vi "MAIN.vi"() -> ()   [LabVIEW 2013]
uses:
  <vilib>/Utility/miscctls.llb/LVRectTypeDef.ctl
  <vilib>/DAQmx/write.llb/DAQmx Write (Analog DBL 1Chan 1Samp).vi
  <vilib>/DAQmx/read.llb/DAQmx Read (Analog 1D DBL NChan 1Samp).vi
  <vilib>/Utility/inputDevices.llb/closeJoystick.vi
  <vilib>/Utility/file.llb/Read From Spreadsheet File (string).vi
  <vilib>/Utility/file.llb/Read From Spreadsheet File (I64).vi
  <vilib>/DAQmx/miscellaneous.llb/DAQmx Fill In Error Info.vi
  <vilib>/Utility/inputDevices.llb/joystickAcquire.vi
panel:
  out "drift_correction_ref":dbl
  out "gpd present":bool
  in  "piezo move":bool=TRUE
  out "device index":i32
  out "read":i64[](array[numeric])
  out "chnl_control":enum16{"MAIN", "QUIT", "INIT", "SAVE"}(ring)=enum."INIT"
  out "state control":T1(ring)=enum."INIT"
  out "channels":string[](array[string])
  out "config":i32[](array[numeric])
  out "Est Power peak":dbl=2.5048715520372213e-09 format="%.4e"
  out "psd":dbl[](graph)
  out "PIEZO":dbl[](graph)
  out "gpd save":bool
  out "gpd start":bool
  out "Tab Control":enum32{"VELO", "KALIB", "channels", "gamepad"}(tab)
  out "Boolean 2":bool
  out "A+B+C+D":dbl format="%#_4f"
  out "(A+B)-(D+C)\n  A+B+C+D":dbl format="%#_4f"
  out "piezo \nposition [nm]":dbl format="%#_4f"
  in  "Z scansize [nm]":i64(slide)=10 min=6000 scale=0.0..6000.0
  in  "Z scanstart [nm]":i64(slide)=10 max=6000 scale=0.0..6000.0
  out "PSD RT":dbl(graph)
  out "first":cluster{"Best Polynomial Fit":dbl[], dbl[]}[](graph)
  in  "SAVE":bool
  in  "start":bool
  out "controls":enum32{"Main controls", "Sub controls"}(tab)
  in  "Advanced":bool
  in  "output folder":path
  in  "multiplier":dbl=10.0
  in  "Gamepad":bool
  in  "kalibruj":bool
  in  "exit":bool
  in  "pause":bool
  in  "slope [nm/V]":dbl format="%.5f"
  in  "pulling speed [nm/s]":dbl=400.0
  in  "Measure\n slope?":bool
  in  "accept calibration":bool
  out "pulling duration [s]":dbl
  in  "piezo movement":enum32{"Radio Selection 1", "Radio Selection 2"}(radio)
  in  "spring constant [N/m]":dbl format="%.5f"
  out "Force [pN]":dbl format="%.2f"
  out "Length [nm]":dbl format="%.2f"
  out "curves count":dbl
  out "saved curves count":i64
  in  "RT DEFLECTION CORRECTION":bool
  in  "deflection correction":bool=TRUE
  in  "alarm":bool=TRUE
  in  "Flip X":bool=TRUE
  in  "Flip Y":bool
  in  "piezo correction hysteresis window [nm]":u32=20
  in  "Drift_crr":bool
  in  "save defaults":bool
  in  "Basic":bool
  in  "spring constatnt\ncorrection factor":dbl=0.817
  in  "samples count/curve":dbl=10000.0 min=100.0 max=1000000.0 step=10000.0
  in  "bcfg":bool
  in  "Terminal_Config":bool
  in  "ambient temp. [Celsius]":dbl=22.0
  in  "auto interval [ms]":u32=1000 max=1000000 step=100
  in  "autosave":bool
  in  "automeasure count":dbl
  in  "auto":bool
  in  "to txt":bool=TRUE
  in  "to datalog":bool=TRUE
  in  "to punias":bool
  out "power peak":dbl
  in  "ponów":bool
  in  "koniec":bool
  in  "stop 2":bool
  in  "Averages":u32(slide)=128 min=64 max=1024 step=64 scale=64.0..1024.0
  out "Spectrum Plot":cluster{dbl, "df":dbl, "Spectrum out":dbl[]}(graph)
  in  "Sampling frequency [Hz]":dbl(slide)=100000.0 step=10000.0 scale=50000.0..150000.0 scale format="%#1_3p"
  in  "Boolean":bool
  in  "piezo sensitivity [nm/V]":dbl=1505.255 format="%#_13g"
  in  "maximum piezo movement range [nm]":i32=6000
  in  "ignore hw error":bool=TRUE
  out "path":path
  in  "SAVE 2":bool
  in  "RELOAD CONFIG":bool
  in  "QUIT":bool
  in  "PIEZO OUTPUT":tag
  in  "PIEZO INPUT":tag
  in  "[(A+B)-(C+D)]/(A+B+C+D)":tag
  in  "A+B+C+D":tag
  in  "gpd_confirm":bool
  in  "device_ok":bool
  out "device name":string
  in  "index":i32
  out "pov 2":bool
  out "pov 3":bool
  out "pov 4":bool
  out "pov 1":bool
  out "button 10":bool
  out "button 9":bool
  out "button 8":bool
  out "button 7":bool
  out "button 6":bool
  out "button 5":bool
  out "button 4":bool
  out "button 3":bool
  out "button 2":bool
  out "button 1":bool
  in  "Ring 14":u16(ring) items=["blank", "speed--", "speed++", "scanstart--", "scanstart++", "scansize--", "scansize++", "x1000", "x100", "x10", "save", "start"]
  in  "Ring 13":u16(ring) items=["blank", "speed--", "speed++", "scanstart--", "scanstart++", "scansize--", "scansize++", "x1000", "x100", "x10", "save", "start"]
  in  "Ring 12":u16(ring) items=["blank", "speed--", "speed++", "scanstart--", "scanstart++", "scansize--", "scansize++", "x1000", "x100", "x10", "save", "start"]
  in  "Ring 8":u16(ring) items=["blank", "speed--", "speed++", "scanstart--", "scanstart++", "scansize--", "scansize++", "x1000", "x100", "x10", "save", "start"]
  in  "Ring 9":u16(ring) items=["blank", "speed--", "speed++", "scanstart--", "scanstart++", "scansize--", "scansize++", "x1000", "x100", "x10", "save", "start"]
  in  "Ring 7":u16(ring) items=["blank", "speed--", "speed++", "scanstart--", "scanstart++", "scansize--", "scansize++", "x1000", "x100", "x10", "save", "start"]
  in  "Ring 11":u16(ring) items=["blank", "speed--", "speed++", "scanstart--", "scanstart++", "scansize--", "scansize++", "x1000", "x100", "x10", "save", "start"]
  in  "Ring 10":u16(ring) items=["blank", "speed--", "speed++", "scanstart--", "scanstart++", "scansize--", "scansize++", "x1000", "x100", "x10", "save", "start"]
  in  "Ring 2":u16(ring) items=["blank", "speed--", "speed++", "scanstart--", "scanstart++", "scansize--", "scansize++", "x1000", "x100", "x10", "save", "start"]
  in  "Ring 4":u16(ring) items=["blank", "speed--", "speed++", "scanstart--", "scanstart++", "scansize--", "scansize++", "x1000", "x100", "x10", "save", "start"]
  in  "Ring 6":u16(ring) items=["blank", "speed--", "speed++", "scanstart--", "scanstart++", "scansize--", "scansize++", "x1000", "x100", "x10", "save", "start"]
  in  "Ring 3":u16(ring) items=["blank", "speed--", "speed++", "scanstart--", "scanstart++", "scansize--", "scansize++", "x1000", "x100", "x10", "save", "start"]
  in  "Ring 5":u16(ring) items=["blank", "speed--", "speed++", "scanstart--", "scanstart++", "scansize--", "scansize++", "x1000", "x100", "x10", "save", "start"]
  in  "Ring":u16(ring) items=["blank", "speed--", "speed++", "scanstart--", "scanstart++", "scansize--", "scansize++", "x1000", "x100", "x10", "save", "start"]
  out "appended array":bool[](array[boolean])
  # "K.Pawlak, J.Strzelecki, Institute of Physics, Nicolaus Copernicus University, Toruñ, Poland"
  # "setup settings"
  # "auto settings"
  # "save formats"
  # "curve"
  # "TERMINAL CONFIGURATION"
  # "1. SELECT PROPER DEVICE"
  # "PREVIEW"
  # "blank\nspeed--\nspeed++\nscanstart--\nscanstart++\nscansize--\nscansize++\nx1000\nx100\nx10\nsave\nstart"
  # "2. CHOOSE BUTTONS FUNCTIONS"
  # "3. CONFIRM BUTTON SETUP"
  # "author K.Pawlak\nInstitute of Physics\nNicolaus Copernicus University\nToruñ, Poland\nAFM gamepad config. ver. 1.0"
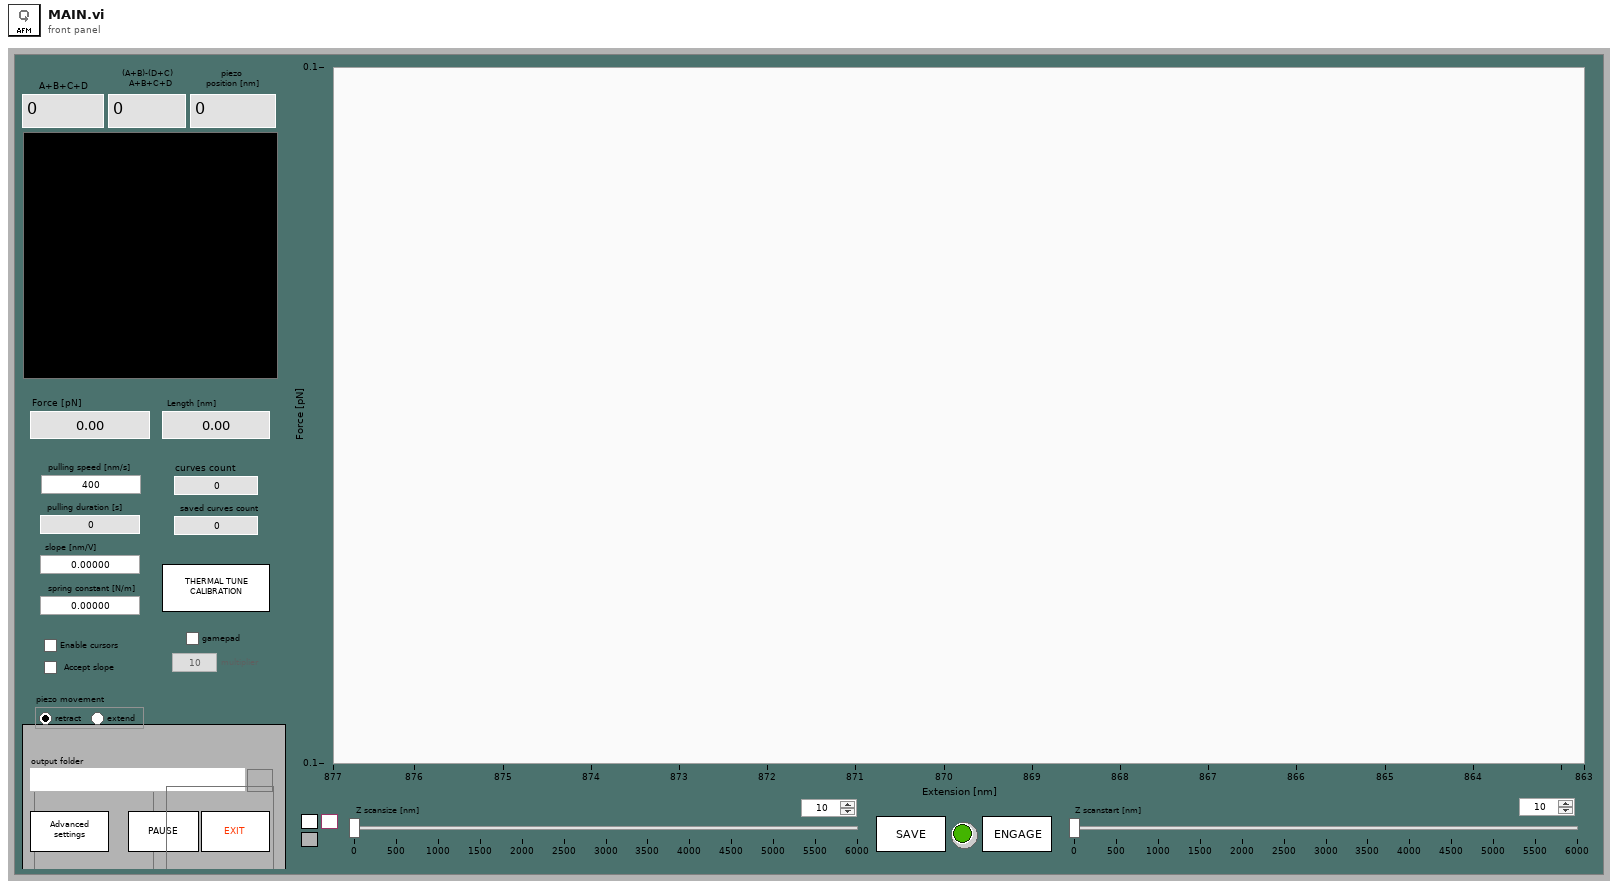
[diagram p1: front panel]
types:
  T1 = enum16{"kalibracja", "INIT", "2", "SAVE", "IDLE", "channels", "pad_cfg"}
  T2 = enum16{"open", "replace", "create", "open or create", "replace or create", "replace or create with confirmation"}
  T3 = enum8{"Enabled", "Disabled", "Disabled and Grayed Out"}
  T4 = typedef "LVRectTypeDef.ctl" = cluster{"Left":i16, "Top":i16, "Right":i16, "Bottom":i16}
  T5 = enum32{"Invalid", "Standard", "Closed", "Hidden", "Minimized", "Maximized"}
  T6 = enum16{"kalibracja", "INIT", "2", "SAVE", "IDLE", "channels"}
  T7 = enum16{"kalibracja", "INIT", "2", "SAVE", "IDLE"}
  T8 = cluster{"PIEZO":dbl[], "psd":dbl[], "Z scanstart [nm]":i64, "slope [nm/V]":dbl, "spring constant [N/m]":dbl, "pulling speed [nm/s]":dbl, "time string":string}
  T9 = cluster{"axes total":u32, "buttons total":u32, "pov total":u32, "device name":string}[]
  T10 = cluster{"axes total":u32, "buttons total":u32, "pov total":u32, "device name":string}
  T11 = cluster{"button 1":bool, "button 2":bool, "button 3":bool, "button 4":bool, "button 5":bool, "button 6":bool, "button 7":bool, "button 8":bool, "button 9":bool, "button 10":bool, "button 11":bool, "button 12":bool, "button 13":bool, "button 14":bool, "button 15":bool, "button 16":bool, "button 17":bool, "button 18":bool, "button 19":bool, "button 20":bool, "button 21":bool, "button 22":bool, "button 23":bool, "button 24":bool, "button 25":bool, "button 26":bool, "button 27":bool, "button 28":bool, "button 29":bool, "button 30":bool, "button 31":bool, "button 32":bool}
  T12 = cluster{"pov 1":i32, "pov 2":i32, "pov 3":i32, "pov 4":i32}
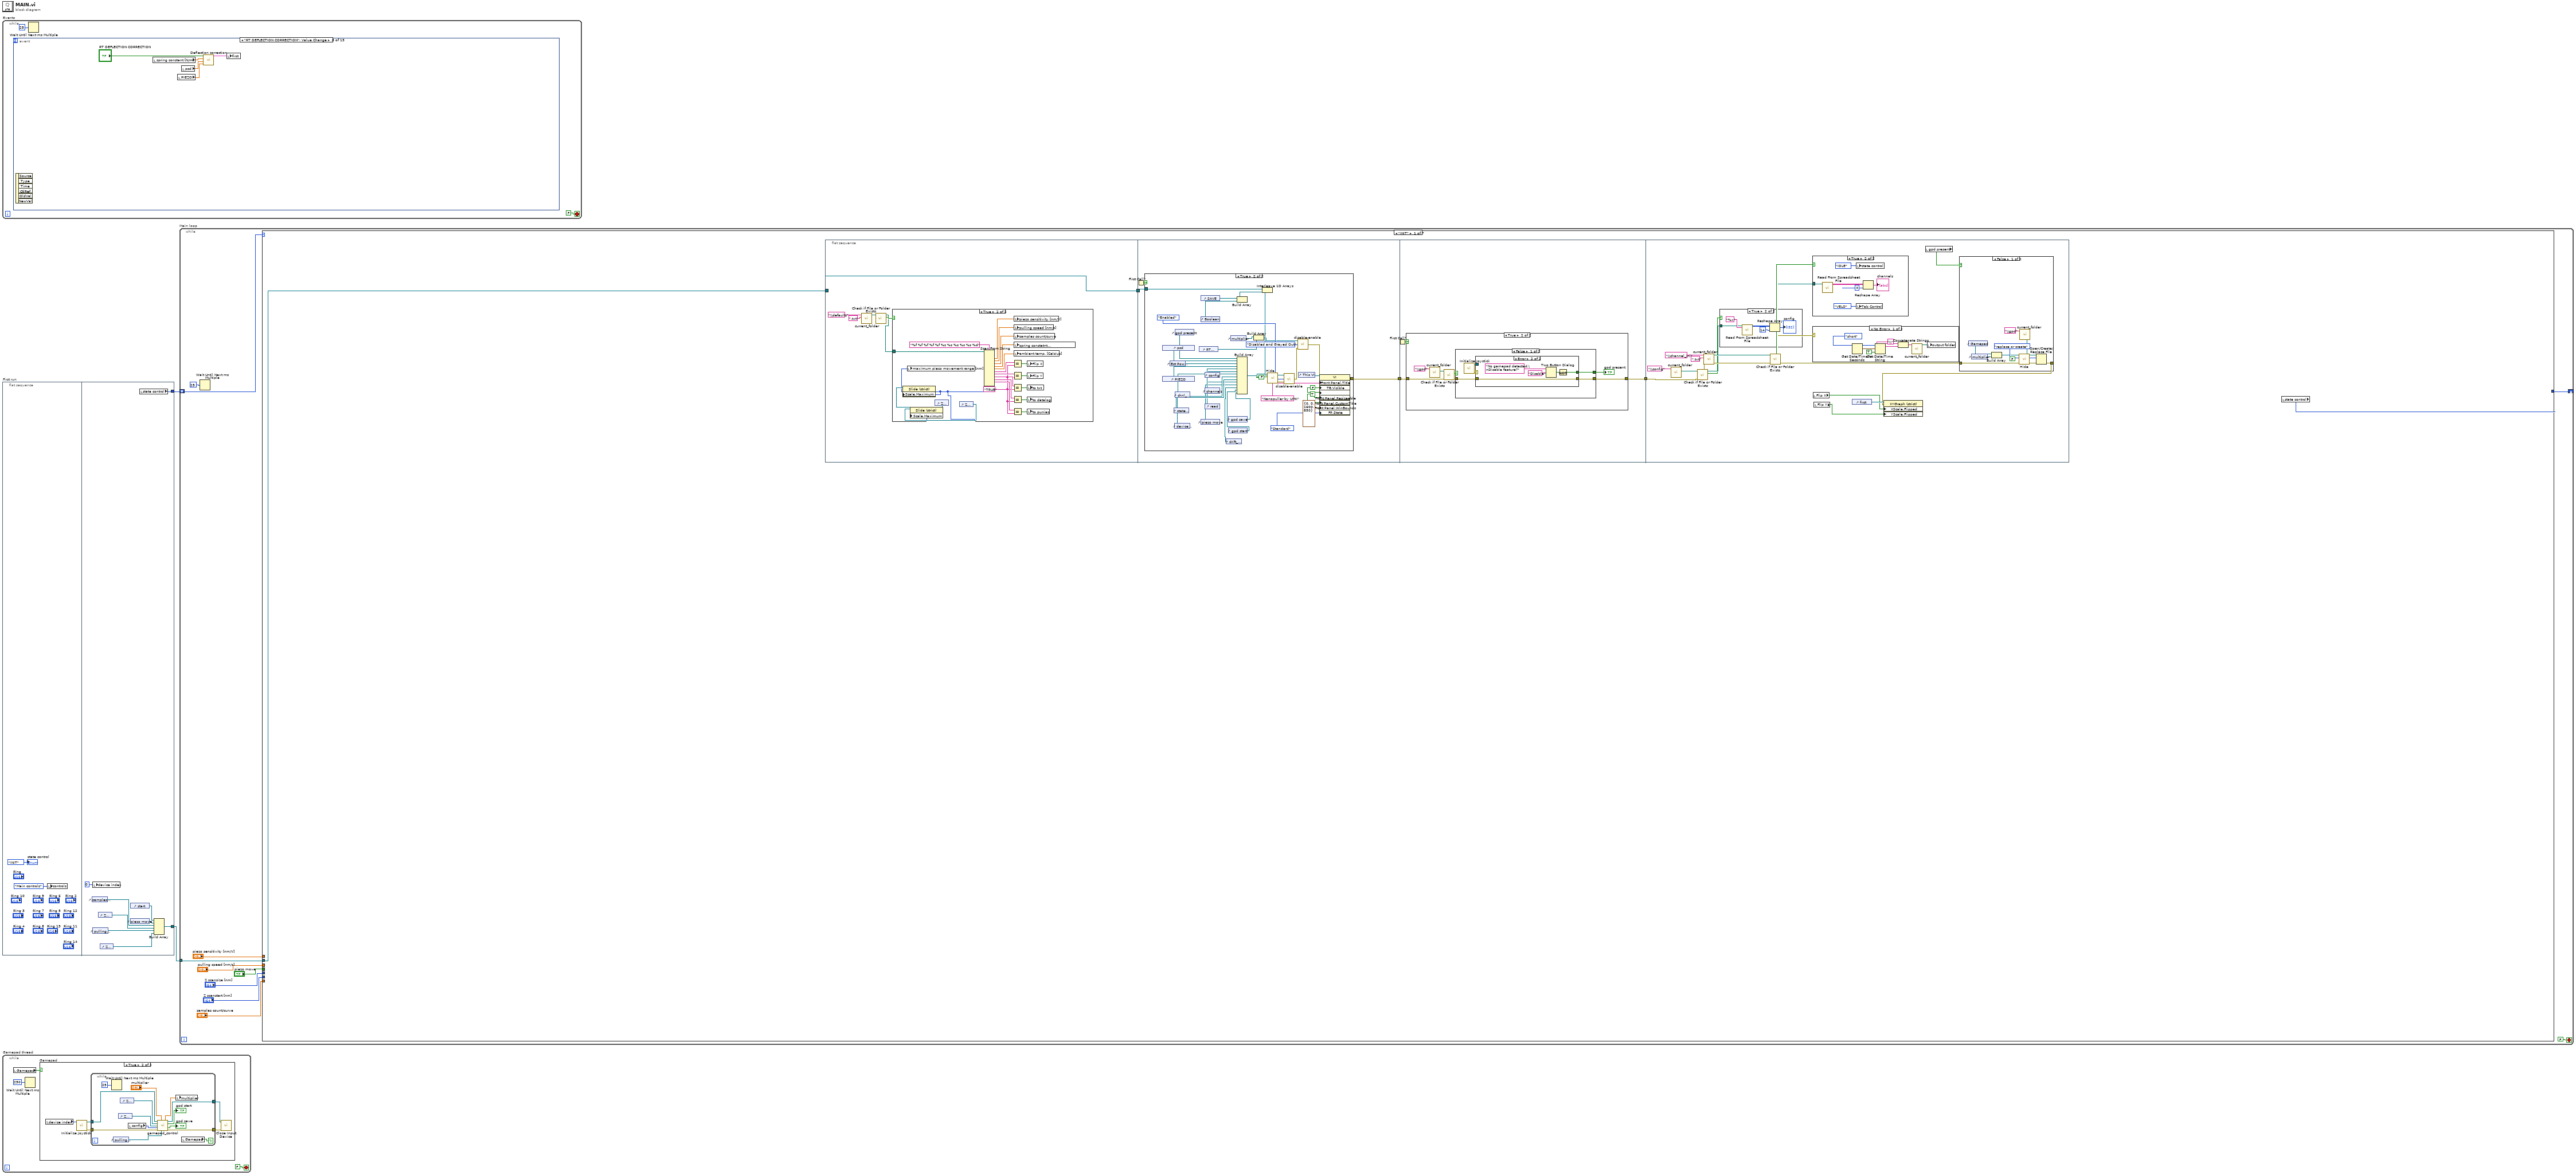
[diagram p0: block diagram]
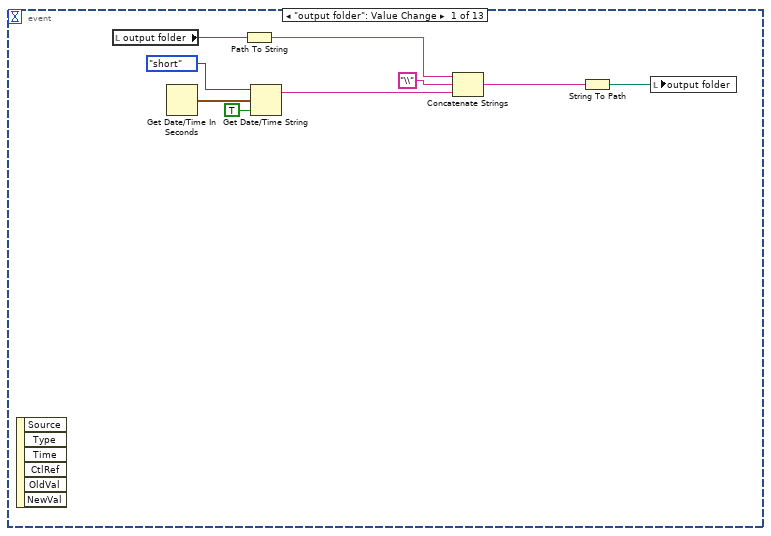
[diagram p3: hidden frame]
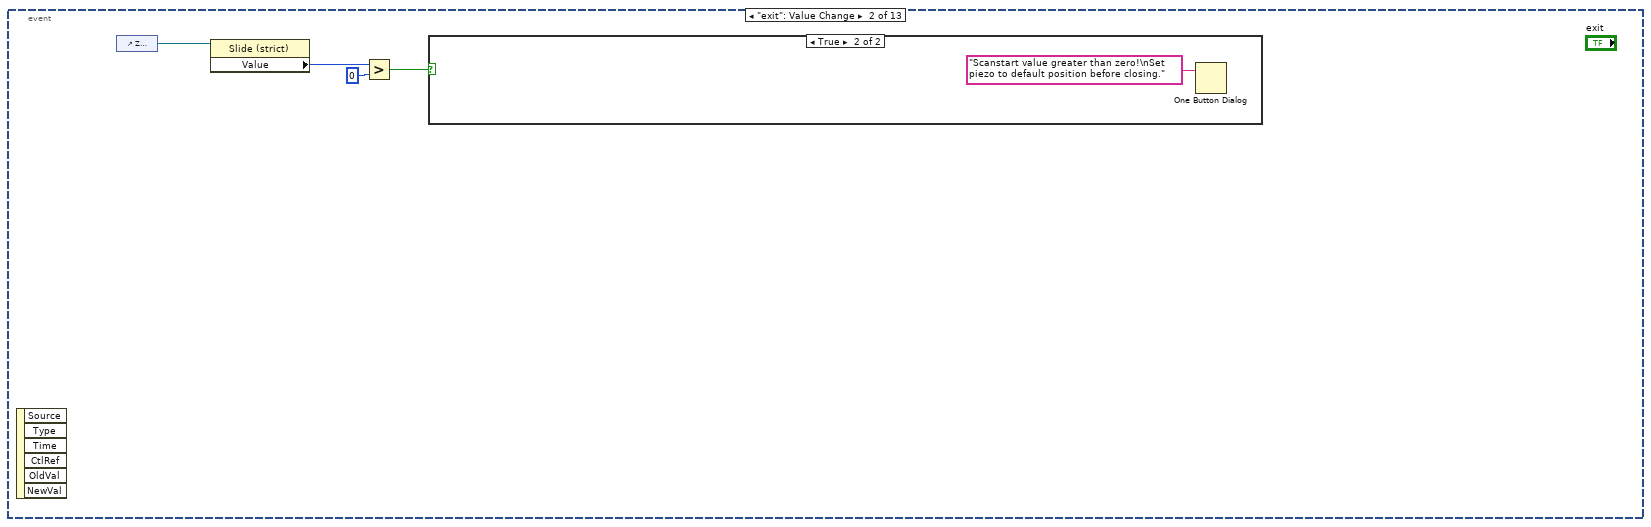
[diagram p4: hidden frame]
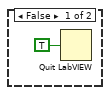
[diagram p5: hidden frame]
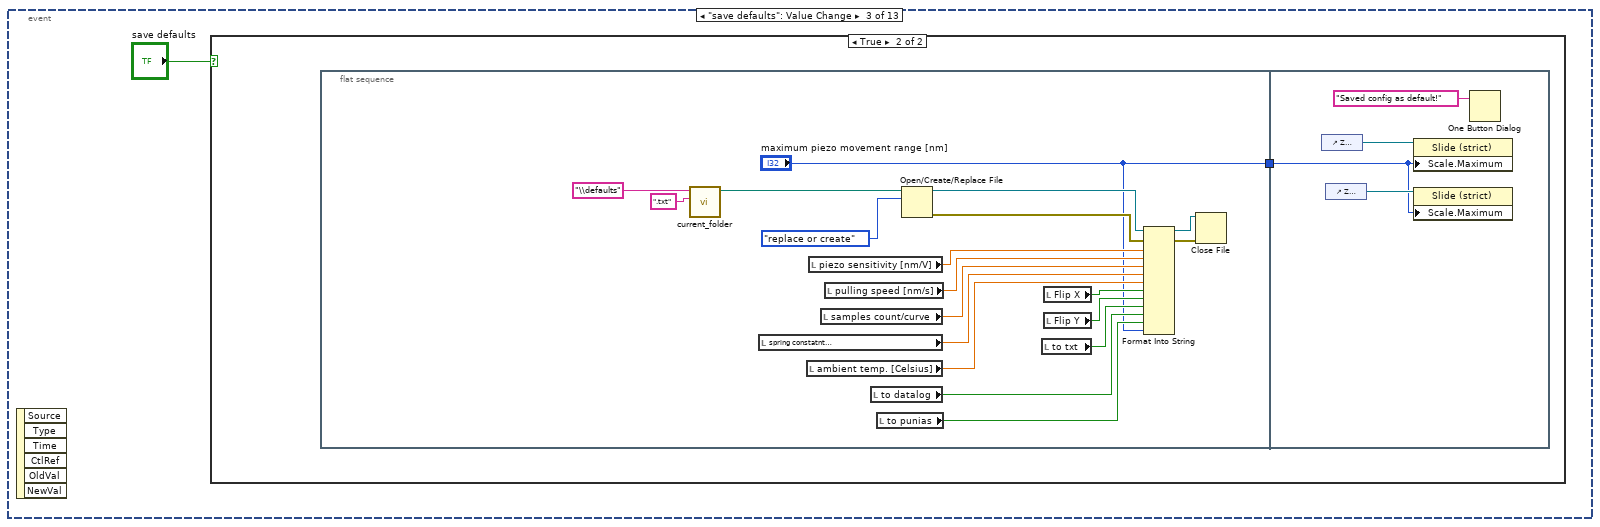
[diagram p6: hidden frame]
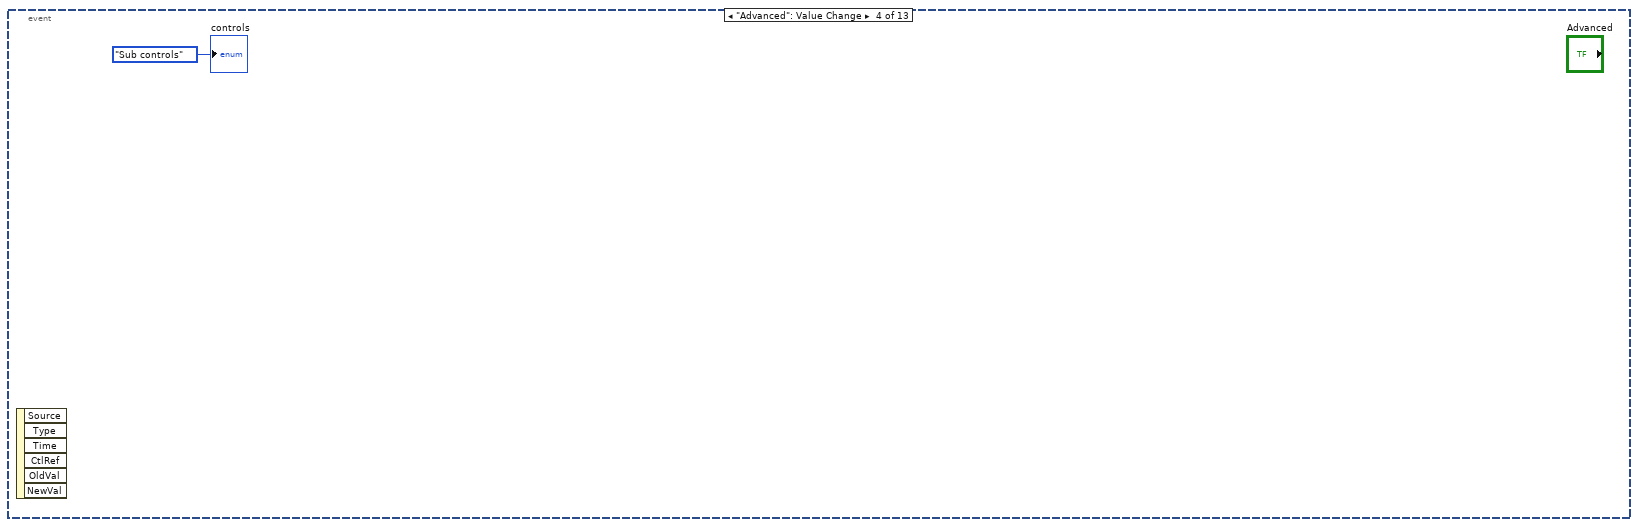
[diagram p8: hidden frame]
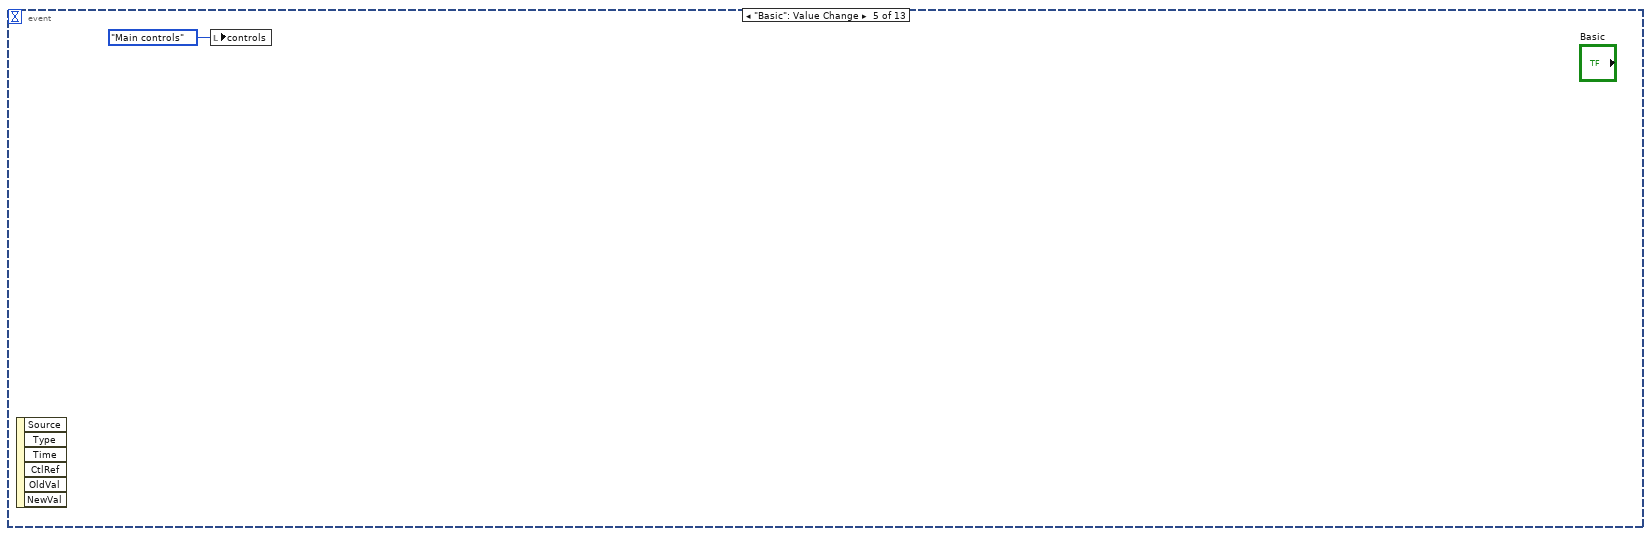
[diagram p9: hidden frame]
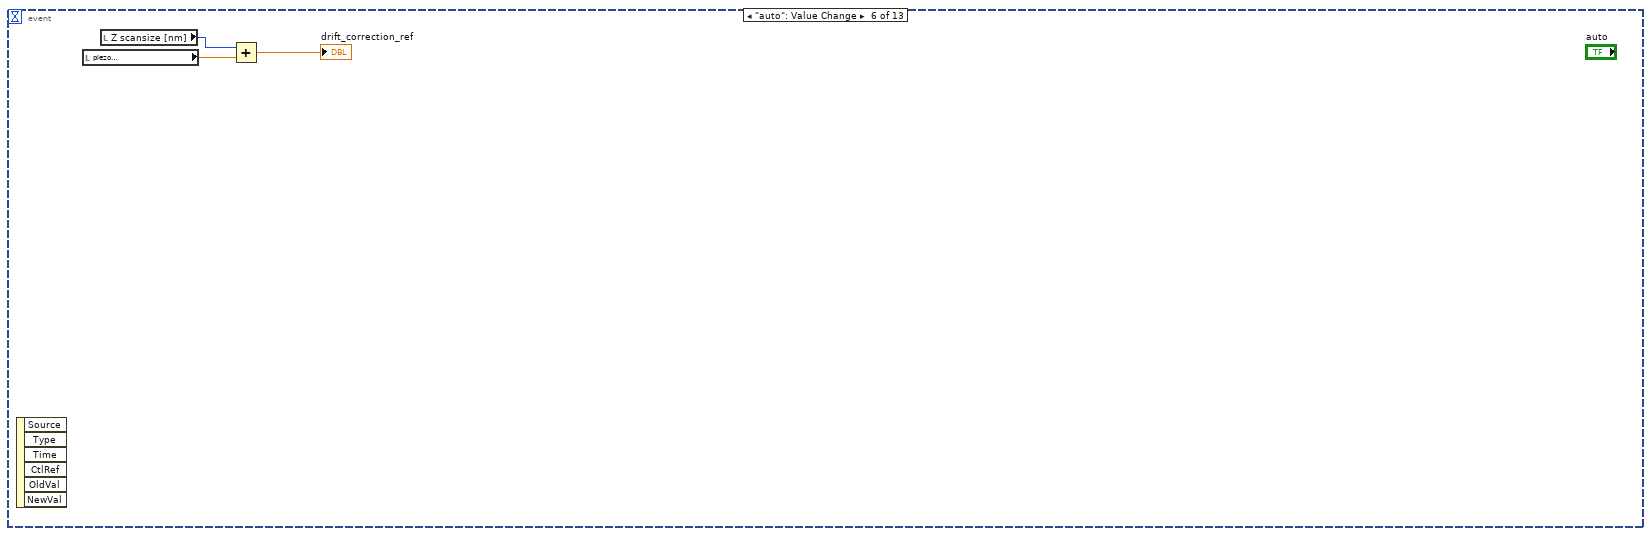
[diagram p10: hidden frame]
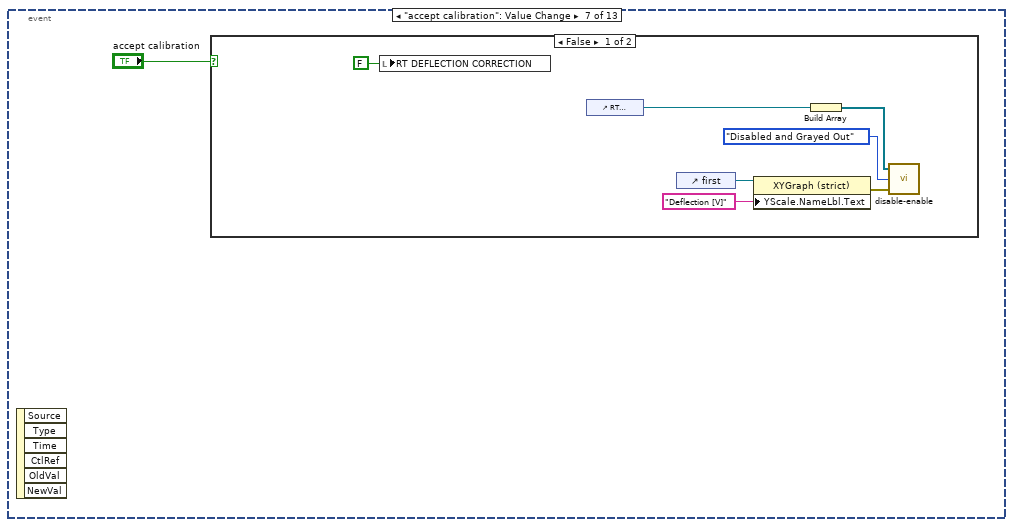
[diagram p11: hidden frame]
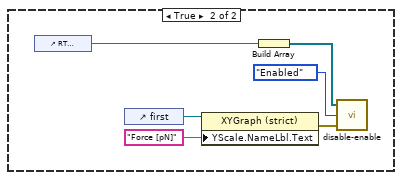
[diagram p12: hidden frame]
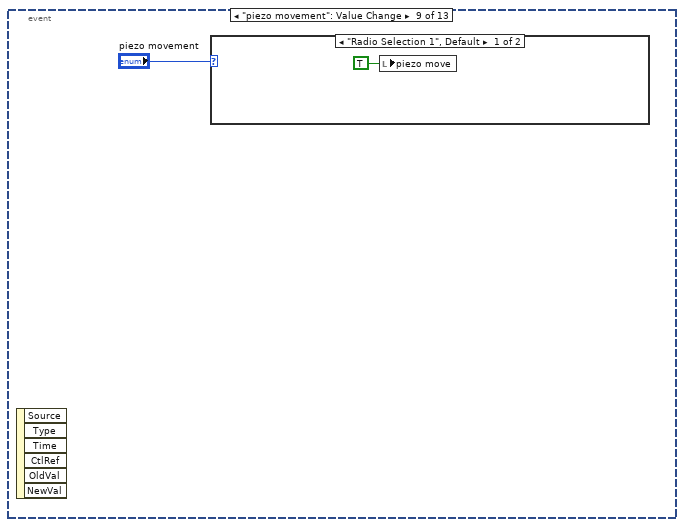
[diagram p13: hidden frame]
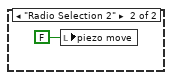
[diagram p14: hidden frame]
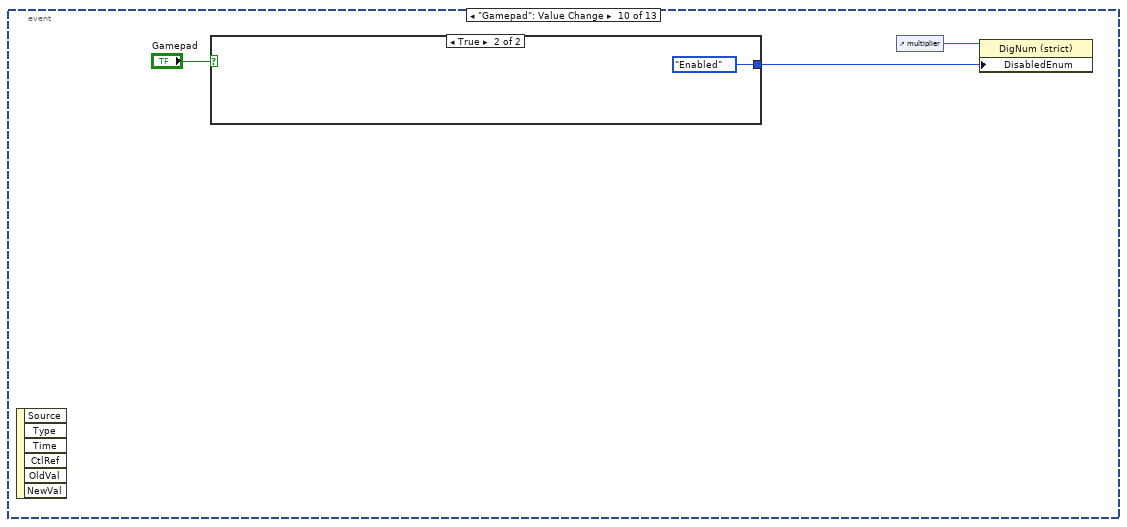
[diagram p15: hidden frame]
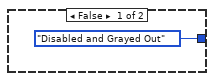
[diagram p16: hidden frame]
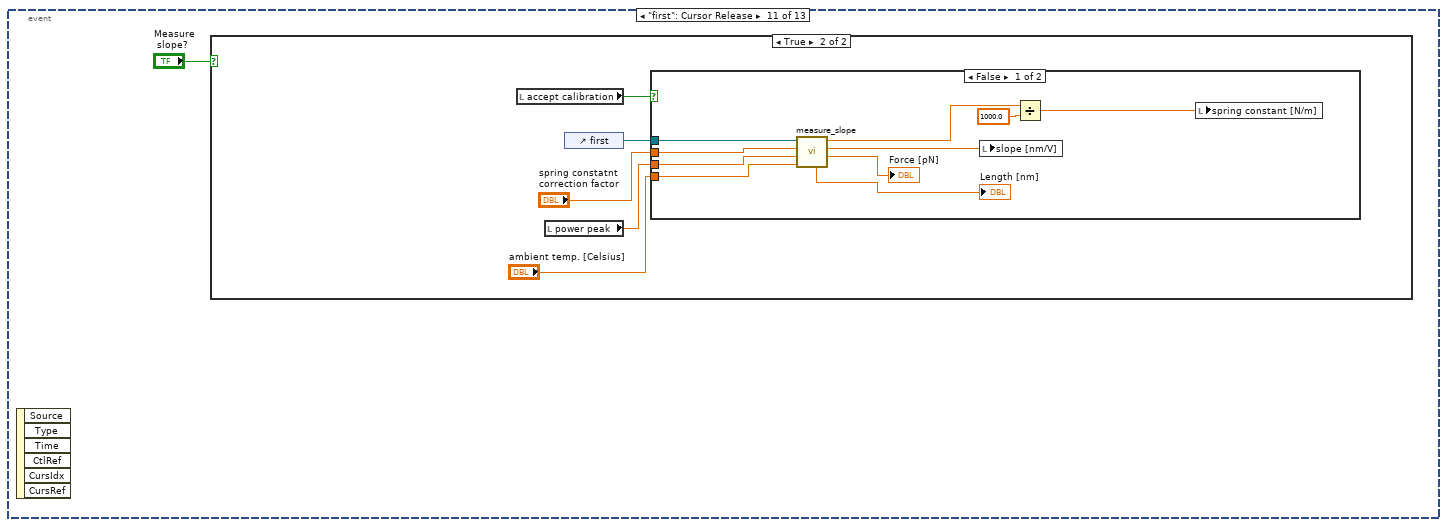
[diagram p17: hidden frame]
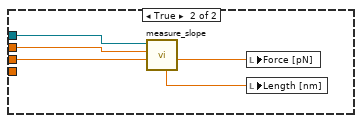
[diagram p19: hidden frame]
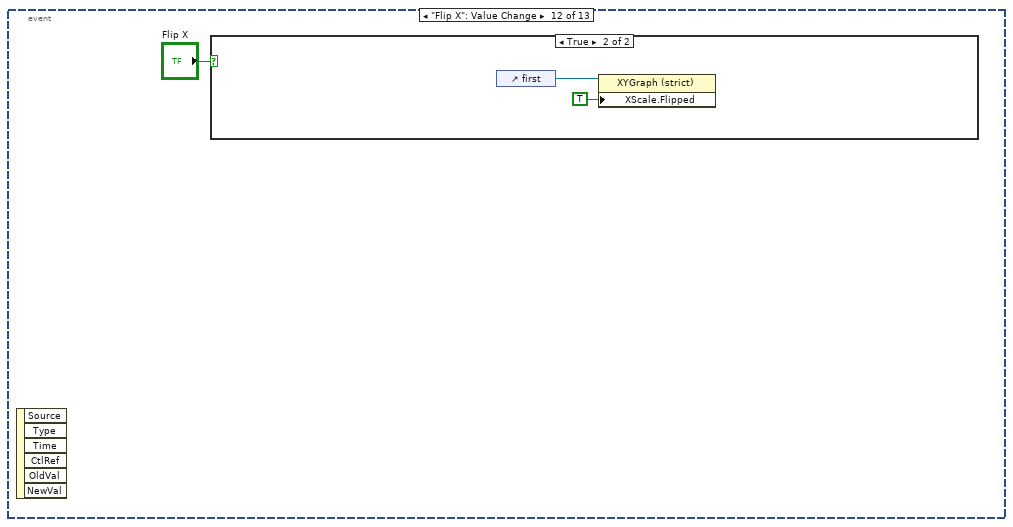
[diagram p20: hidden frame]
diagram:
  n1 = while "Events" {
    stop <- FALSE stop-if-true
    n2 = event shown="[7] \"RT DEFLECTION CORRECTION\": Value Change" {
      selector: _ -> [_ _ _ _ _ _ _ _ _ _ _ _ _]
      dyn-events: _ -> [_ _ _ _ _ _ _ _ _ _ _ _ _]
      timeout: _ -> [_ _ _ _ _ _ _ _ _ _ _ _ _]
      event "output folder": Value Change {
        n3 = event-data() -> ()  [unwired: 1 in, 6 out]
        n4 = local read "output folder"() -> (w10:path)
        n5 = Get Date/Time In Seconds() -> (seconds since 1Jan1904=w12:timestamp)
        n6 = Path To String(path=w10) -> (string=w9:string)
        n7 = Get Date/Time String(date format (0)=enum16{"short", "long", "abbreviated"}."short", seconds (now)=w12, want seconds? (F)=TRUE) -> (date string=w6:string)  [unwired: 1 out]
        n8 = Concatenate Strings(w9, "\\" ("string"), w6) -> (w7:string)
        n9 = String To Path(string=w7) -> (path=w8:path)
        n10 = local write "output folder"(w8) -> ()
      }
      event "exit": Value Change {
        n11 = event-data() -> ()  [unwired: 1 in, 6 out]
        n12 = control-ref of="Z scanstart [nm]"() -> (w15:refnum<vi>)
        n13 = property class="Slide (strict)"(reference=w15) -> ("Value"=w16:i64)  [unwired: 1 in, 2 out]
        n14 = Greater?(x=w16, y=i64 0) -> (0:w14:bool)
        n15 = case shown="True" w14 {
          frame False {
            n16 = Quit LabVIEW(quit? (T)=TRUE) -> ()
          }
          frame True {
            n17 = One Button Dialog(message="Scanstart value greater than zero!\nSet piezo to default position before closing.") -> ()  [unwired: 1 in, 1 out]
          }
        }
      }
      event "save defaults": Value Change {
        n18 = event-data() -> ()  [unwired: 1 in, 6 out]
        n19 = case shown="True" "save defaults" {
          frame False {
          }
          frame True {
            n20 = flat-sequence {
              tunnel: ["maximum piezo movement range [nm]"] -> w21
              tunnel: w21 -> [w41]
              frame #0 {
                n21 = call "current_folder.vi"("extension"=".txt", "filename"="\\defaults") -> ("Path"=w30:path)  [unwired: 9 in]
                n22 = local read "spring constatnt\ncorrection factor"() -> (w33:dbl)
                n23 = local read "ambient temp. [Celsius]"() -> (w32:dbl)
                n24 = local read "piezo sensitivity [nm/V]"() -> (w36:dbl)
                n25 = local read "samples count/curve"() -> (w34:dbl)
                n26 = local read "pulling speed [nm/s]"() -> (w35:dbl)
                n27 = local read "to datalog"() -> (w24:bool)
                n28 = local read "to punias"() -> (w23:bool)
                n29 = Open/Create/Replace File(file path (use dialog)=w30, operation (0:open)=T2."replace or create") -> (refnum out=w29:refnum<file>, error out=w26:errorcluster)  [unwired: 4 in, 1 out]
                n30 = local read "to txt"() -> (w25:bool)
                n31 = local read "Flip X"() -> (w39:bool)
                n32 = local read "Flip Y"() -> (w38:bool)
                n33 = Format Into String(initial string=w29, error in=w26, w36, w35, w34, w33, w32, w39, w38, w25, w24, w23, "maximum piezo movement range [nm]") -> (resulting string=w28:refnum<file>, error out=w27:errorcluster)  [unwired: 1 in]
                n34 = Close File(refnum=w28, error in=w27) -> ()  [unwired: 2 out]
              }
              frame #1 {
                n35 = control-ref of="Z scanstart [nm]"() -> (w42:refnum<vi>)
                n36 = control-ref of="Z scansize [nm]"() -> (w43:refnum<vi>)
                n37 = property class="Slide (strict)"(reference=w42, "Scale.Maximum"=w41) -> ()  [unwired: 1 in, 2 out]
                n38 = property class="Slide (strict)"(reference=w43, "Scale.Maximum"=w41) -> ()  [unwired: 1 in, 2 out]
                n39 = One Button Dialog(message="Saved config as default!") -> ()  [unwired: 1 in, 1 out]
              }
            }
          }
        }
      }
      event "Advanced": Value Change {
        n40 = event-data() -> ()  [unwired: 1 in, 6 out]
        "controls" <- enum32{"Main controls", "Sub controls"}."Sub controls" ("controls")
      }
      event "Basic": Value Change {
        n41 = event-data() -> ()  [unwired: 1 in, 6 out]
        n42 = local write "controls"(enum32{"Main controls", "Sub controls"}."Main controls" ("controls")) -> ()
      }
      event "auto": Value Change {
        n43 = event-data() -> ()  [unwired: 1 in, 6 out]
        n44 = local read "piezo \nposition [nm]"() -> (w48:dbl)
        n45 = local read "Z scansize [nm]"() -> (w49:i64)
        n46 = Add(x=w49, y=w48) -> (x+y=→"drift_correction_ref":dbl)
      }
      event "accept calibration": Value Change {
        n47 = event-data() -> ()  [unwired: 1 in, 6 out]
        n48 = case shown="False" "accept calibration" {
          frame False {
            n49 = local write "RT DEFLECTION CORRECTION"(FALSE ("RT DEFLECTION CORRECTION")) -> ()
            n50 = control-ref of="RT DEFLECTION CORRECTION"() -> (w55:refnum<vi>)
            n51 = control-ref of="first"() -> (w57:refnum<vi>)
            n52 = property class="XYGraph (strict)"(reference=w57, "YScale.NameLbl.Text"="Deflection [V]" ("X Scale.Name Label.Text")) -> (error out=w52:errorcluster)  [unwired: 1 in, 1 out]
            n53 = Build Array(w55) -> (w54:refnum<vi>[])
            n54 = call "disable-enable.vi"("error in (no error)"=w52, "Disabled"=T3."Disabled and Grayed Out", "Array"=w54) -> ()  [unwired: 1 out]
          }
          frame True {
            n55 = control-ref of="RT DEFLECTION CORRECTION"() -> (w61:refnum<vi>)
            n56 = control-ref of="first"() -> (w63:refnum<vi>)
            n57 = property class="XYGraph (strict)"(reference=w63, "YScale.NameLbl.Text"="Force [pN]" ("X Scale.Name Label.Text")) -> (error out=w58:errorcluster)  [unwired: 1 in, 1 out]
            n58 = Build Array(w61) -> (w60:refnum<vi>[])
            n59 = call "disable-enable.vi"("error in (no error)"=w58, "Disabled"=T3."Enabled", "Array"=w60) -> ()  [unwired: 1 out]
          }
        }
      }
      event "RT DEFLECTION CORRECTION": Value Change {
        n60 = event-data() -> ()  [unwired: 1 in, 6 out]
        n61 = local read "spring constant [N/m]"() -> (w67:dbl)
        n62 = local read "PIEZO"() -> (w65:dbl[])
        n63 = local read "psd"() -> (w66:dbl[])
        n64 = call "Deflection correction.vi"("fitted piezo"=w65, "psd"=w66, "spring constant [N/m]"=w67, "RT DEFLECTION CORRECTION"="RT DEFLECTION CORRECTION") -> ("Array"=w64:cluster{dbl[], dbl[]}[])  [unwired: 7 in]
        n65 = local write "first"(w64) -> ()
      }
      event "piezo movement": Value Change {
        n66 = event-data() -> ()  [unwired: 1 in, 6 out]
        n67 = case shown="\"Radio Selection 1\", Default" "piezo movement" {
          frame "Radio Selection 1", Default {
            n68 = local write "piezo move"(TRUE ("piezo move")) -> ()
          }
          frame "Radio Selection 2" {
            n69 = local write "piezo move"(FALSE ("piezo move")) -> ()
          }
        }
      }
      event "Gamepad": Value Change {
        n70 = event-data() -> ()  [unwired: 1 in, 6 out]
        n71 = case shown="True" "Gamepad" {
          tunnel: [T3."Disabled and Grayed Out" ("Disabled") T3."Enabled" ("Disabled")] -> w73
          frame False {
          }
          frame True {
          }
        }
        n72 = control-ref of="multiplier"() -> (w74:refnum<vi>)
        n73 = property class="DigNum (strict)"(reference=w74, "DisabledEnum"=w73) -> ()  [unwired: 1 in, 2 out]
      }
      event "first": Cursor Release {
        n74 = event-data() -> ()  [unwired: 1 in, 6 out]
        n75 = case shown="True" "Measure\n slope?" {
          frame False {
          }
          frame True {
            n76 = local read "accept calibration"() -> (w79:bool)
            n77 = local read "power peak"() -> (w80:dbl)
            n78 = control-ref of="first"() -> (w82:refnum<vi>)
            n79 = case shown="False" w79 {
              tunnel: w82 -> [w92 w95]
              tunnel: "spring constatnt\ncorrection factor" -> [w91 w94]
              tunnel: w80 -> [w90 w93]
              tunnel: "ambient temp. [Celsius]" -> [w85 _]
              frame False {
                n80 = call "measure_slope.vi"("temp"=w85, "power peak"=w90, "correction factor"=w91, "XYGraph in"=w92) -> ("Numeric 3"=→"Force [pN]":dbl, "Numeric 2"=w84:dbl, "Numeric"=w86:dbl, "Numeric 4"=→"Length [nm]":dbl)  [unwired: 4 in]
                n81 = local write "slope [nm/V]"(w84) -> ()
                n82 = Divide(x=w86, y=1000.0) -> (x/y=w83:dbl)
                n83 = local write "spring constant [N/m]"(w83) -> ()
              }
              frame True {
                n84 = call "measure_slope.vi"("power peak"=w93, "correction factor"=w94, "XYGraph in"=w95) -> ("Numeric 3"=w97:dbl, "Numeric 4"=w96:dbl)  [unwired: 5 in, 2 out]
                n85 = local write "Force [pN]"(w97) -> ()
                n86 = local write "Length [nm]"(w96) -> ()
              }
            }
          }
        }
      }
      event "Flip X": Value Change {
        n87 = event-data() -> ()  [unwired: 1 in, 6 out]
        n88 = case shown="True" "Flip X" {
          frame False {
            n89 = control-ref of="first"() -> (w100:refnum<vi>)
            n90 = property class="XYGraph (strict)"(reference=w100, "XScale.Flipped"=FALSE ("X Scale.Flipped")) -> ()  [unwired: 1 in, 2 out]
          }
          frame True {
            n91 = control-ref of="first"() -> (w102:refnum<vi>)
            n92 = property class="XYGraph (strict)"(reference=w102, "XScale.Flipped"=TRUE ("X Scale.Flipped")) -> ()  [unwired: 1 in, 2 out]
          }
        }
      }
      event "Flip Y": Value Change {
        n93 = event-data() -> ()  [unwired: 1 in, 6 out]
        n94 = case shown="False" "Flip Y" {
          frame False {
            n95 = control-ref of="first"() -> (w105:refnum<vi>)
            n96 = property class="XYGraph (strict)"(reference=w105, "YScale.Flipped"=FALSE ("Y Scale.Flipped")) -> ()  [unwired: 1 in, 2 out]
          }
          frame True {
            n97 = control-ref of="first"() -> (w107:refnum<vi>)
            n98 = property class="XYGraph (strict)"(reference=w107, "YScale.Flipped"=TRUE ("Y Scale.Flipped")) -> ()  [unwired: 1 in, 2 out]
          }
        }
      }
    }
    n99 = Wait Until Next ms Multiple(millisecond multiple=u32 25) -> ()  [unwired: 1 out]
  }
  n100 = flat-sequence "First run" {
    tunnel: [w112] -> w2
    tunnel: [w111] -> w1
    frame #0 {
      n101 = local write "controls"(enum32{"Main controls", "Sub controls"}."Main controls" ("controls")) -> ()
      "state control" <- T1."INIT" ("state control")
    }
    frame #1 {
      n102 = control-ref of="samples count/curve"() -> (w115:refnum<vi>)
      n103 = control-ref of="pulling speed [nm/s]"() -> (w117:refnum<vi>)
      n104 = local write "device index"(0 ("device index")) -> ()
      n105 = control-ref of="Z scanstart [nm]"() -> (w116:refnum<vi>)
      n106 = control-ref of="Z scansize [nm]"() -> (w118:refnum<vi>)
      n107 = control-ref of="start"() -> (w113:refnum<vi>)
      n108 = control-ref of="piezo move"() -> (w114:refnum<vi>)
      n109 = local read "state control"() -> (w111:T1)
      n110 = Build Array(w113, w114, w115, w116, w117, w118) -> (w112:refnum<vi>[])
    }
  }
  n111 = while "Gamepad thread" {
    stop <- FALSE stop-if-true
    n112 = local read "Gamepad"() -> (w121:bool)
    n113 = Wait Until Next ms Multiple(millisecond multiple=u32 250) -> ()  [unwired: 1 out]
    n114 = case "Gamepad" shown="True" w121 {
      frame False {
      }
      frame True {
        n115 = local read "device index"() -> (w123:i32)
        n116 = call <vilib>:"Initialize Joystick.vi"("device index"=w123) -> ("error out"=w122:errorcluster, "device ID"=w126:refnum<k1>)  [unwired: 9 in]
        n117 = while {
          tunnel: w122 -> [w130]
          tunnel: w126 -> [w129]
          tunnel: [w128] -> w125
          tunnel: [w127] -> w124
          stop <- w134 continue-if-true
          n118 = Wait Until Next ms Multiple(millisecond multiple=u32 25) -> ()  [unwired: 1 out]
          n119 = control-ref of="pulling speed [nm/s]"() -> (w136:refnum<vi>)
          n120 = control-ref of="Z scanstart [nm]"() -> (w139:refnum<vi>)
          n121 = control-ref of="Z scansize [nm]"() -> (w140:refnum<vi>)
          n122 = local read "config"() -> (w135:i32[])
          n123 = call "gamepad_control.vi"("device ID in"=w129, "preskaler 2"="multiplier", "scansize [nm]"=w140, "scanstart [nm]"=w139, "read"=w135, "error in (no error)"=w130, "dynamika [nm/s]"=w136) -> ("preskaler"=w137:dbl, "Refnum out"=w128:refnum<k1>, "START"=→"gpd start":bool, "SAVE"=→"gpd save":bool, "error out"=w127:errorcluster)  [unwired: 3 in, 1 out]
          n124 = local write "multiplier"(w137) -> ()
          n125 = local read "Gamepad"() -> (w134:bool)
        }
        n126 = call-poly <vilib>:"Close Input Device.vi"("error in (no error)"=w124, "device ID"=w125) -> ()  [unwired: 8 in, 1 out]
      }
    }
  }
  n127 = while "Main loop" {
    tunnel: w2 -> [w151]
    shift-right: [w144] -> _
    shift-left: w1 -> [w145]
    stop <- FALSE stop-if-true
    n128 = Wait Until Next ms Multiple(millisecond multiple=u32 25 ("milliseconds to wait")) -> ()  [unwired: 1 out]
    n129 = case shown="\"INIT\"" w145 {
      tunnel: w151 -> [w156 w327 _ w550 _ _ _]
      tunnel: "Z scansize [nm]" -> [_ _ _ w552 _ _ _]
      tunnel: "pulling speed [nm/s]" -> [_ _ _ w548 _ _ _]
      tunnel: "Z scanstart [nm]" -> [_ _ _ w549 _ _ _]
      tunnel: "samples count/curve" -> [_ _ _ w547 _ _ _]
      tunnel: "piezo move" -> [_ _ _ w551 _ _ _]
      tunnel: [w155 w313 T7."IDLE" ("Enum 2") w546 w610 T1."INIT" ("state control") w891] -> w144
      tunnel: "piezo sensitivity [nm/V]" -> [_ w326 _ w545 _ _ _]
      frame "INIT" {
        n130 = flat-sequence {
          tunnel: w156 -> [w162]
          tunnel: [w162] -> w152
          tunnel: [w194] -> w154
          tunnel: w152 -> [w195]
          tunnel: w154 -> [w233]
          tunnel: [w232] -> w153
          tunnel: w153 -> [w265]
          frame #0 {
            n131 = call "current_folder.vi"("extension"=".txt", "filename"="\\defaults") -> ("Path"=w159:path)  [unwired: 9 in]
            n132 = call <vilib>:"Check if File or Folder Exists.vi"("path"=w159) -> ("file or folder exists?"=w158:bool, "dup path"=w157:path)  [unwired: 8 in, 1 out]
            n133 = case shown="True" w158 {
              tunnel: w157 -> [_ w187]
              frame False {
                n134 = control-ref of="ambient temp. [Celsius]"() -> (w165:refnum<vi>)
                n135 = control-ref of="piezo sensitivity [nm/V]"() -> (w170:refnum<vi>)
                n136 = control-ref of="samples count/curve"() -> (w168:refnum<vi>)
                n137 = control-ref of="pulling speed [nm/s]"() -> (w169:refnum<vi>)
                n138 = control-ref of="spring constatnt\ncorrection factor"() -> (w166:refnum<vi>)
                n139 = control-ref of="Flip X"() -> (w164:refnum<vi>)
                n140 = control-ref of="Flip Y"() -> (w163:refnum<vi>)
                n141 = Build Array(w170, w169, w168, w166, w165, w164, w163) -> (w167:refnum<vi>[])
                n142 = for {
                  tunnel: w167 -> [w171] mode=indexing
                  n143 = invoke class="Ctl" method="Reinit To Default"(reference=w171) -> ()  [unwired: 2 in, 3 out]
                }
              }
              frame True {
                w178 = "TRUE" ("y")
                n144 = control-ref of="Z scanstart [nm]"() -> (w174:refnum<vi>)
                n145 = control-ref of="Z scansize [nm]"() -> (w173:refnum<vi>)
                n146 = Scan From String("%f %f %f %f %f %s %s %s %s %s %d" ("format string"), w187) -> (output 1=w186:dbl, output 2=w185:dbl, output 3=w184:dbl, output 4=w183:dbl, output 5=w182:dbl, output 6=w191:string, output 7=w190:string, output 8=w181:string, output 9=w180:string, output 10=w179:string, output 11=w172:i32)  [unwired: 12 in, 2 out]
                n147 = property class="Slide (strict)"(reference=w174, "Scale.Maximum"=w172) -> ()  [unwired: 1 in, 2 out]
                n148 = local write "maximum piezo movement range [nm]"(w172) -> ()
                n149 = property class="Slide (strict)"(reference=w173, "Scale.Maximum"=w172) -> ()  [unwired: 1 in, 2 out]
                n150 = Equal?(x=w191, y=w178) -> (x = y?=w189:bool)
                n151 = Equal?(x=w190, y=w178) -> (x = y?=w188:bool)
                n152 = Equal?(x=w181, y=w178) -> (x = y?=w177:bool)
                n153 = Equal?(x=w180, y=w178) -> (x = y?=w176:bool)
                n154 = Equal?(x=w179, y=w178) -> (x = y?=w175:bool)
                n155 = local write "piezo sensitivity [nm/V]"(w186) -> ()
                n156 = local write "pulling speed [nm/s]"(w185) -> ()
                n157 = local write "samples count/curve"(w184) -> ()
                n158 = local write "spring constatnt\ncorrection factor"(w183) -> ()
                n159 = local write "ambient temp. [Celsius]"(w182) -> ()
                n160 = local write "Flip X"(w189) -> ()
                n161 = local write "Flip Y"(w188) -> ()
                n162 = local write "to txt"(w177) -> ()
                n163 = local write "to datalog"(w176) -> ()
                n164 = local write "to punias"(w175) -> ()
              }
            }
          }
          frame #1 {
            n165 = First Call?() -> (First Call?: T/F=w193:bool)
            n166 = case shown="True" w193 {
              tunnel: w195 -> [_ w228]
              tunnel: [_ w210] -> w194
              frame False {
              }
              frame True {
                w206 = FALSE ("Front Panel Window:Show Menu Bar")
                n167 = control-ref of="psd"() -> (w221:refnum<vi>)
                n168 = control-ref of="PIEZO"() -> (w222:refnum<vi>)
                n169 = control-ref of="Est Power peak"() -> (w225:refnum<vi>)
                n170 = control-ref of="state control"() -> (w216:refnum<vi>)
                n171 = control-ref of="device index"() -> (w215:refnum<vi>)
                n172 = control-ref of="gpd present"() -> (w205:refnum<vi>)
                n173 = control-ref of="chnl_control"() -> (w217:refnum<vi>)
                n174 = control-ref of="RT DEFLECTION CORRECTION"() -> (w196:refnum<vi>)
                n175 = control-ref of="SAVE"() -> (w231:refnum<vi>)
                n176 = control-ref of="Boolean"() -> (w226:refnum<vi>)
                n177 = control-ref of="piezo move"() -> (w213:refnum<vi>)
                n178 = control-ref of="config"() -> (w219:refnum<vi>)
                n179 = control-ref of="channels"() -> (w218:refnum<vi>)
                n180 = control-ref of="read"() -> (w214:refnum<vi>)
                n181 = control-ref of="drift_correction_ref"() -> (w198:refnum<vi>)
                n182 = control-ref of="gpd save"() -> (w199:refnum<vi>)
                n183 = control-ref of="gpd start"() -> (w197:refnum<vi>)
                n184 = control-ref of="multiplier"() -> (w202:refnum<vi>)
                n185 = Build Array(w231, w226) -> (w229:refnum<vi>[])
                n186 = Build Array(w205, w221, w225, w222, w219, w218, w217, w216, w215, w214, w213, w198, w197, w199) -> (w224:refnum<vi>[])
                n187 = Build Array(w202, w196) -> (w201:refnum<vi>[])
                n188 = Interleave 1D Arrays(w228, w229) -> (w227:refnum<vi>[])
                n189 = call "Hide.vi"("Visible"=FALSE, "Array"=w224) -> ("error out"=w223:errorcluster)  [unwired: 9 in]
                n190 = call "disable-enable.vi"("error in (no error)"=w223, "Disabled"=T3."Enabled", "Array"=w227) -> ("error out"=w204:errorcluster)
                n191 = call "disable-enable.vi"("error in (no error)"=w204, "Disabled"=T3."Disabled and Grayed Out", "Array"=w201) -> ("error out"=w203:errorcluster)
                n192 = control-ref of="This VI"() -> (w211:refnum<vi>)
                n193 = property class="VI"(reference=w211, error in=w203, "Front Panel.Title"="Nanopuller by UMK" ("Front Panel Window:Title"), "TB.Visible"=w206, "Front Panel.ShowMenuBar"=w206, "Front Panel.Resizeable"=w206, "Front Panel.CustomTitle"=TRUE ("Front Panel Window:Keep Window Proportions"), "Front Panel.WinBounds"=T4 {"Left"=0, "Top"=0, "Right"=1600, "Bottom"=850} ("Front Panel Window:Window Bounds"), "FP.State"=T5."Standard" ("Front Panel Window:State")) -> (error out=w210:errorcluster)  [unwired: 1 out]
              }
            }
          }
          frame #2 {
            n194 = First Call?() -> (First Call?: T/F=w234:bool)
            n195 = case shown="True" w234 {
              tunnel: w233 -> [w235 w237]
              tunnel: [w235 w242] -> w232
              frame False {
              }
              frame True {
                n196 = call "current_folder.vi"("filename"="\\gpd") -> ("Path"=w241:path)  [unwired: 10 in]
                n197 = call <vilib>:"Check if File or Folder Exists.vi"("error in (no error)"=w237, "path"=w241) -> ("error out"=w236:errorcluster, "file or folder exists?"=w239:bool)  [unwired: 7 in, 1 out]
                n198 = case shown="False" w239 {
                  tunnel: w236 -> [w247 w257]
                  tunnel: [w246 w257] -> w242
                  tunnel: [w243 FALSE ("T button?")] -> w238
                  frame False {
                    n199 = call <vilib>:"Initialize Joystick.vi"() -> ("error out"=w244:errorcluster, "device ID"=w245:refnum<k1>)  [unwired: 10 in]
                    n200 = case shown="Error" w244 {
                      selector: w244 -> [w248 _]
                      tunnel: [TRUE ("T button?") w252] -> w243
                      tunnel: w247 -> [w249 w254]
                      tunnel: [w249 w254] -> w246
                      tunnel: w245 -> [w250 _]
                      frame No Error {
                        n201 = call-poly <vilib>:"Close Input Device.vi"("error in (no error)"=w248, "device ID"=w250) -> ()  [unwired: 8 in, 1 out]
                      }
                      frame Error {
                        n202 = Two Button Dialog(message="No gamepad detected.\nDisable feature?", 2:"Disable" ("T button name (\"OK\")")) -> (T button?=w253:bool)  [unwired: 1 in]
                        n203 = Not(x=w253) -> (.not. x?=w252:bool)
                      }
                    }
                  }
                  frame True {
                  }
                }
                "gpd present" <- w238
              }
            }
          }
          frame #3 {
            n204 = call "current_folder.vi"("filename"="\\config") -> ("Path"=w275:path)  [unwired: 10 in]
            n205 = call <vilib>:"Check if File or Folder Exists.vi"("error in (no error)"=w265, "path"=w275) -> ("error out"=w273:errorcluster, "file or folder exists?"=w266:bool, "dup path"=w267:path)  [unwired: 7 in]
            n206 = call "current_folder.vi"("extension"=".txt", "filename"="\\channel_ini") -> ("Path"=w269:path)  [unwired: 9 in]
            n207 = case shown="True" w266 {
              tunnel: w267 -> [_ w308]
              frame False {
              }
              frame True {
                n208 = call-poly <vilib>:"Read From Spreadsheet File.vi"("format (%d)"="%x", "file path (dialog if empty)"=w308) -> ("all rows"=w309:i64[][])  [unwired: 5 in, 4 out]
                n209 = Reshape Array(w309, 14 ("dimension size")) -> (→"config":i64[])
              }
            }
            n210 = call <vilib>:"Check if File or Folder Exists.vi"("error in (no error)"=w273, "path"=w269) -> ("error out"=w263:errorcluster, "file or folder exists?"=w272:bool, "dup path"=w268:path)  [unwired: 7 in]
            n211 = case shown="True" w272 {
              tunnel: w268 -> [_ w307]
              frame False {
                n212 = local write "chnl_control"(enum16{"MAIN", "QUIT", "INIT", "SAVE"}."INIT" ("chnl_control")) -> ()
                n213 = local write "Tab Control"(enum32{"VELO", "KALIB", "channels"}."channels" ("Tab Control")) -> ()
                n214 = local write "state control"(T6."channels" ("state control")) -> ()
              }
              frame True {
                n215 = call-poly <vilib>:"Read From Spreadsheet File.vi"("file path (dialog if empty)"=w307) -> ("all rows"=w304:string[][])  [unwired: 6 in, 4 out]
                n216 = local write "state control"(T6."IDLE" ("state control")) -> ()
                n217 = local write "Tab Control"(enum32{"VELO", "KALIB", "channels"}."VELO" ("Tab Control")) -> ()
                n218 = Reshape Array(w304, 4 ("dimension size")) -> (→"channels":string[])
              }
            }
            n219 = case shown="No Error" w263 {
              frame No Error {
                n220 = Get Date/Time In Seconds() -> (seconds since 1Jan1904=w297:timestamp)
                n221 = Get Date/Time String(date format (0)=enum16{"short", "long", "abbreviated"}."short", seconds (now)=w297, want seconds? (F)=TRUE) -> (date string=w293:string)  [unwired: 1 out]
                n222 = Concatenate Strings("\\" ("string"), w293) -> (w292:string)
                n223 = call "current_folder.vi"("filename"=w292) -> ("Path"=w298:path)  [unwired: 10 in]
                n224 = local write "output folder"(w298) -> ()
              }
              frame Error {
              }
            }
            n225 = local read "Flip X"() -> (w260:bool)
            n226 = local read "Flip Y"() -> (w259:bool)
            n227 = control-ref of="first"() -> (w262:refnum<vi>)
            n228 = local read "gpd present"() -> (w264:bool)
            n229 = case shown="False" w264 {
              tunnel: w263 -> [w277 w287]
              tunnel: [w276 w286] -> w261
              frame False {
                n230 = control-ref of="Gamepad"() -> (w280:refnum<vi>)
                n231 = control-ref of="multiplier"() -> (w279:refnum<vi>)
                n232 = Build Array(w280, w279) -> (w282:refnum<vi>[])
                n233 = call "Hide.vi"("error in (no error)"=w277, "Visible"=FALSE, "Array"=w282) -> ("error out"=w278:errorcluster)  [unwired: 8 in]
                n234 = call "current_folder.vi"("filename"="\\gpd") -> ("Path"=w284:path)  [unwired: 10 in]
                n235 = Open/Create/Replace File(file path (use dialog)=w284, error in=w278, operation (0:open)=T2."replace or create") -> (error out=w276:errorcluster)  [unwired: 3 in, 2 out]
              }
              frame True {
                n236 = control-ref of="Gamepad"() -> (w289:refnum<vi>)
                n237 = control-ref of="multiplier"() -> (w288:refnum<vi>)
                n238 = Build Array(w288, w289) -> (w291:refnum<vi>[])
                n239 = call "Hide.vi"("error in (no error)"=w287, "Visible"=TRUE, "Array"=w291) -> ("error out"=w286:errorcluster)  [unwired: 8 in]
              }
            }
            n240 = property class="XYGraph (strict)"(reference=w262, error in=w261, "XScale.Flipped"=w260, "YScale.Flipped"=w259) -> ()  [unwired: 2 out]
          }
        }
        n241 = local read "state control"() -> (w155:T1)
      }
      frame "IDLE" {
        n242 = local write "state control"(T6."IDLE" ("state control")) -> ()
        n243 = local read "channels"() -> (w324:string[])
        n244 = call "disable-enable.vi"("Array"=w327) -> ("error out"=w316:errorcluster)  [unwired: 2 in]
        n245 = call "init_idle_channels.vi"("channels"=w324, "error in"=w316) -> ("Refnum out"=w323:refnum<k21>, "task out"=w321:refnum<k21>, "error out"=w322:errorcluster)  [unwired: 1 in]
        n246 = while {
          tunnel: w326 -> [w369]
          tunnel: [w383] -> w314
          tunnel: w323 -> [w378]
          tunnel: w322 -> [w340]
          tunnel: w321 -> [w373]
          tunnel: [w366] -> w320
          tunnel: [w365] -> w318
          tunnel: ["pause"] -> w315
          stop <- w361 stop-if-true
          n247 = local read "Z scanstart [nm]"() -> (w352:i64)
          n248 = local read "Z scansize [nm]"() -> (w351:i64)
          n249 = Greater?(x=w351, y=w352) -> (0:w356:bool)
          n250 = case shown="True" "ignore hw error" {
            tunnel: [w392 w394] -> w341
            tunnel: w340 -> [w392 w393]
            frame False {
            }
            frame True {
              n251 = call <vilib>:"Clear Errors.vi"("error in (no error)"=w393) -> ("error out"=w394:errorcluster)  [unwired: 6 in]
            }
          }
          n252 = local read "Z scanstart [nm]"() -> (w379:i64)
          n253 = local read "piezo move"() -> (w353:bool)
          n254 = Divide(x=w379, y=w369) -> (x/y=w380:dbl)
          n255 = And(x=w356, y=w353) -> (x .and. y?=w358:bool)
          n256 = Equal?(x=w351, y=i64 0) -> (x = y?=w359:bool)
          n257 = Or(x=w358, y=w359) -> (x .or. y?=w355:bool)
          n258 = call-poly <vilib>:"DAQmx Write.vi"("task/channels in"=w378, "data"=w380, "error in"=w341) -> ("task out"=w366:refnum<k21>, "error out"=w374:errorcluster)  [unwired: 10 in, 1 out]
          n259 = case shown="True" w355 {
            tunnel: [T3."Enabled" ("Disabled") T3."Disabled and Grayed Out" ("Disabled")] -> w346
            frame False {
            }
            frame True {
            }
          }
          n260 = call-poly <vilib>:"DAQmx Read.vi"("task/channels in"=w373, "error in"=w374) -> ("task out"=w365:refnum<k21>, "data"=w372:dbl[], "error out"=w339:errorcluster)  [unwired: 11 in]
          n261 = case shown="False" "ignore hw error" {
            tunnel: w339 -> [w389 w391]
            tunnel: [w389 w390] -> w338
            frame False {
            }
            frame True {
              n262 = call <vilib>:"Clear Errors.vi"("error in (no error)"=w391) -> ("error out"=w390:errorcluster)  [unwired: 6 in]
            }
          }
          n263 = control-ref of="auto"() -> (w347:refnum<vi>)
          n264 = Index Array(array=w372, index #1=0 ("index"), index #2=1 ("length"), index #3=2 ("index")) -> (element #1=→"A+B+C+D":dbl, element #2=→"PSD RT" →"(A+B)-(D+C)\n  A+B+C+D":dbl, element #3=w370:dbl)
          n265 = property class="Bool (strict)"(reference=w347, error in=w338, "DisabledEnum"=w346) -> (error out=w345:errorcluster)  [unwired: 1 out]
          n266 = control-ref of="start"() -> (w354:refnum<vi>)
          n267 = Multiply(x=w370, y=w369) -> (x*y=→"piezo \nposition [nm]":dbl)
          n268 = property class="Bool"(reference=w354, error in=w345, "DisabledEnum"=w346) -> (error out=w343:errorcluster)  [unwired: 1 out]
          n269 = local read "auto"() -> (w334:bool)
          n270 = case "Auto" shown="True" w334 {
            tunnel: [FALSE ("autosave") w401] -> w348
            tunnel: w343 -> [w398 w400]
            tunnel: [w398 w400] -> w344
            frame False {
            }
            frame True {
              n271 = flat-sequence {
                tunnel: [w456] -> w401
                frame #0 {
                  n272 = Wait (ms)(milliseconds to wait="auto interval [ms]") -> ()  [unwired: 1 out]
                }
                frame #1 {
                  n273 = case shown="True" "Drift_crr" {
                    frame False {
                    }
                    frame True {
                      n274 = local read "piezo movement"() -> (w405:enum32{"Radio Selection 1", "Radio Selection 2"})
                      n275 = case shown="\"Radio Selection 2\"" w405 {
                        tunnel: "piezo correction hysteresis window [nm]" -> [w408 w433]
                        frame "Radio Selection 1", Default {
                          n276 = local read "piezo \nposition [nm]"() -> (w416:dbl)
                          n277 = local read "drift_correction_ref"() -> (w413:dbl)
                          n278 = local read "Z scansize [nm]"() -> (w417:i64)
                          n279 = Divide(x=w408, y=2.0) -> (x/y=w411:dbl)
                          n280 = Add(x=w411, y=w413) -> (x+y=w410:dbl)
                          n281 = Subtract(x=w413, y=w411) -> (x-y=w412:dbl)
                          n282 = Add(x=w417, y=w416) -> (x+y=w409:dbl)
                          n283 = control-ref of="Z scansize [nm]"() -> (w407:refnum<vi>)
                          n284 = Greater?(x=w409, y=w410) -> (0:w414:bool)
                          n285 = Less?(x=w409, y=w412) -> (x < y?=w415:bool)
                          n286 = property class="Slide (strict)"(reference=w407) -> ("Scale.Maximum"=w406:dbl)  [unwired: 1 in, 2 out]
                          n287 = case shown="True" w414 {
                            tunnel: w411 -> [_ w427]
                            tunnel: w406 -> [_ w425]
                            frame False {
                            }
                            frame True {
                              n288 = local read "Z scanstart [nm]"() -> (w430:i64)
                              n289 = local read "Z scansize [nm]"() -> (w426:i64)
                              n290 = Subtract(x=w430, y=w427) -> (x-y=w429:dbl)
                              n291 = In Range and Coerce(upper limit=w425, x=w429, lower limit=w426) -> (coerced(x)=w428:dbl)  [unwired: 1 out]
                              n292 = local write "Z scanstart [nm]"(w428) -> ()
                            }
                          }
                          n293 = case shown="True" w415 {
                            tunnel: w411 -> [_ w421]
                            tunnel: w406 -> [_ w419]
                            frame False {
                            }
                            frame True {
                              n294 = local read "Z scanstart [nm]"() -> (w424:i64)
                              n295 = local read "Z scansize [nm]"() -> (w420:i64)
                              n296 = Add(x=w421, y=w424) -> (x+y=w423:dbl)
                              n297 = In Range and Coerce(upper limit=w419, x=w423, lower limit=w420) -> (coerced(x)=w422:dbl)  [unwired: 1 out]
                              n298 = local write "Z scanstart [nm]"(w422) -> ()
                            }
                          }
                        }
                        frame "Radio Selection 2" {
                          n299 = local read "piezo \nposition [nm]"() -> (w441:dbl)
                          n300 = local read "drift_correction_ref"() -> (w438:dbl)
                          n301 = local read "Z scansize [nm]"() -> (w442:i64)
                          n302 = Divide(x=w433, y=2.0) -> (x/y=w436:dbl)
                          n303 = control-ref of="Z scansize [nm]"() -> (w432:refnum<vi>)
                          n304 = Add(x=w436, y=w438) -> (x+y=w435:dbl)
                          n305 = Subtract(x=w438, y=w436) -> (x-y=w437:dbl)
                          n306 = Add(x=w442, y=w441) -> (x+y=w434:dbl)
                          n307 = property class="Slide (strict)"(reference=w432) -> ("Scale.Maximum"=w431:dbl)  [unwired: 1 in, 2 out]
                          n308 = Greater?(x=w434, y=w435) -> (0:w439:bool)
                          n309 = Less?(x=w434, y=w437) -> (x < y?=w440:bool)
                          n310 = case shown="True" w439 {
                            tunnel: w436 -> [_ w451]
                            tunnel: w431 -> [_ w450]
                            frame False {
                            }
                            frame True {
                              n311 = local read "Z scanstart [nm]"() -> (w455:i64)
                              n312 = Subtract(x=w455, y=w451) -> (x-y=w453:dbl)
                              n313 = In Range and Coerce(upper limit=w450, x=w453, lower limit=0.0) -> (coerced(x)=w452:dbl)  [unwired: 1 out]
                              n314 = local write "Z scanstart [nm]"(w452) -> ()
                            }
                          }
                          n315 = case shown="True" w440 {
                            tunnel: w436 -> [_ w445]
                            tunnel: w431 -> [_ w444]
                            frame False {
                            }
                            frame True {
                              n316 = local read "Z scanstart [nm]"() -> (w449:i64)
                              n317 = Add(x=w445, y=w449) -> (x+y=w447:dbl)
                              n318 = In Range and Coerce(upper limit=w444, x=w447, lower limit=0.0) -> (coerced(x)=w446:dbl)  [unwired: 1 out]
                              n319 = local write "Z scanstart [nm]"(w446) -> ()
                            }
                          }
                        }
                      }
                    }
                  }
                }
                frame #2 {
                  n320 = Greater?(x="automeasure count", y=0.0) -> (0:w457:bool)
                  n321 = case shown="False" w457 {
                    tunnel: [w461 TRUE ("y")] -> w456
                    frame False {
                      w461 = FALSE ("autosave")
                      n322 = case shown="True" "alarm" {
                        frame False {
                        }
                        frame True {
                          n323 = call <vilib>:"Beep.vi"() -> ()  [unwired: 12 in]
                        }
                      }
                      n324 = local write "auto"(w461) -> ()
                      n325 = local write "autosave"(w461) -> ()
                    }
                    frame True {
                      n326 = local read "automeasure count"() -> (w465:dbl)
                      n327 = Decrement(x=w465) -> (x-1=w464:dbl)
                      n328 = local write "automeasure count"(w464) -> ()
                      n329 = local write "autosave"(TRUE ("autosave")) -> ()
                    }
                  }
                }
              }
            }
          }
          n330 = case "HW errors" shown="Error" w343 {
            tunnel: [FALSE ("true") w396] -> w342
            frame No Error {
            }
            frame Error {
              n331 = One Button Dialog(message="Invalid device configuration!") -> (true=w396:bool)  [unwired: 1 in]
            }
          }
          n332 = Or(x="start", y=w348) -> (x .or. y?=w349:bool)
          n333 = local read "gpd start"() -> (w336:bool)
          n334 = local read "gpd save"() -> (w335:bool)
          n335 = call "case_selector.vi"("kalibruj"="kalibruj", "Terminal_Config"="Terminal_Config", "bcfg in"="bcfg", "SAVE"="SAVE", "start in"=w349, "SAVE 2"=w335, "error in (no error)"=w344, "START"=w336) -> ("Boolean 3"=w387:bool, "Boolean 2"=w385:bool, "start out"=w384:bool, "bcfg out"=w381:bool, "Boolean"=w382:bool)  [unwired: 3 in]
          n336 = case "Case select" shown="False" w381 {
            tunnel: w387 -> [w475 _]
            tunnel: w385 -> [w474 _]
            tunnel: w384 -> [w473 _]
            tunnel: [w472 TRUE ("START")] -> w362
            tunnel: [w471 T1."pad_cfg" ("Enum 2")] -> w383
            tunnel: w382 -> [w470 _]
            tunnel: "Terminal_Config" -> [w469 _]
            tunnel: w342 -> [w468 _]
            frame False {
              n337 = case shown="False" w475 {
                tunnel: [w481 w495] -> w471
                tunnel: w474 -> [_ w494]
                tunnel: w470 -> [_ _]
                tunnel: [w480 TRUE ("START")] -> w472
                tunnel: w473 -> [w479 _]
                tunnel: w469 -> [w478 _]
                tunnel: w468 -> [w476 _]
                frame False {
                  n338 = Or(x=w478, y=w476) -> (x .or. y?=w477:bool)
                  n339 = case shown="True" w477 {
                    tunnel: [w484 T6."channels" ("Enum 2")] -> w481
                    tunnel: [w482 TRUE ("START")] -> w480
                    tunnel: w479 -> [w483 _]
                    frame False {
                      n340 = case shown="False" w483 {
                        tunnel: [T7."IDLE" ("Enum 2") T7."2" ("Enum 2")] -> w484
                        tunnel: [FALSE ("START") TRUE ("START")] -> w482
                        frame False {
                        }
                        frame True {
                        }
                      }
                    }
                    frame True {
                      n341 = local write "Tab Control"(enum32{"VELO", "KALIB", "channels"}."channels" ("Tab Control")) -> ()
                      "chnl_control" <- enum16{"MAIN", "QUIT", "INIT", "SAVE"}."INIT" ("chnl_control")
                    }
                  }
                }
                frame True {
                  n342 = case shown="False" w494 {
                    tunnel: [T7."kalibracja" ("Enum 2") T7."SAVE" ("Enum 2")] -> w495
                    frame False {
                    }
                    frame True {
                    }
                  }
                }
              }
            }
            frame True {
              n343 = local write "Tab Control"(enum32{"VELO", "KALIB", "channels", "gamepad"}."gamepad" ("Tab Control")) -> ()
              n344 = local write "state control"(T1."pad_cfg" ("state control")) -> ()
            }
          }
          n345 = Or(x=w362, y="pause") -> (x .or. y?=w361:bool)
        }
        n346 = case "Pause/empty loop" shown="True" w315 {
          tunnel: w314 -> [w328 w330]
          tunnel: [w328 w329] -> w313
          frame False {
          }
          frame True {
            n347 = while {
              tunnel: w330 -> [w333]
              tunnel: [w333] -> w329
              stop <- w332 continue-if-true
              n348 = local read "pause"() -> (w332:bool)
              n349 = Wait Until Next ms Multiple(millisecond multiple=u32 250) -> ()  [unwired: 1 out]
            }
          }
        }
        n350 = call <vilib>:"DAQmx Clear Task.vi"("task in"=w320) -> ("error out"=w319:errorcluster)  [unwired: 14 in]
        n351 = call <vilib>:"DAQmx Clear Task.vi"("task in"=w318, "error in"=w319) -> ("error out"=w317:errorcluster)  [unwired: 13 in]
        n352 = call <vilib>:"Clear Errors.vi"("error in (no error)"=w317) -> ()  [unwired: 6 in, 1 out]
      }
      frame "SAVE" {
        n353 = flat-sequence {
          frame #0 {
            w513 = "_"
            n354 = First Call?() -> (First Call?: T/F=w510:bool)
            n355 = case shown="False" w510 {
              tunnel: [w530 1 ("device index")] -> w509
              frame False {
                n356 = local read "saved curves count"() -> (w531:i64)
                n357 = Increment(x=w531) -> (x+1=w530:i64)
              }
              frame True {
              }
            }
            "saved curves count" <- w509
            n358 = local read "pulling speed [nm/s]"() -> (w516:dbl)
            n359 = local read "spring constant [N/m]"() -> (w519:dbl)
            n360 = Get Date/Time In Seconds() -> (seconds since 1Jan1904=w527:timestamp)
            n361 = local read "Z scanstart [nm]"() -> (w521:i64)
            n362 = local read "slope [nm/V]"() -> (w520:dbl)
            n363 = local read "PIEZO"() -> (w522:dbl[])
            n364 = Path To String(path="output folder") -> (string=w524:string)
            n365 = local read "psd"() -> (w515:dbl[])
            n366 = Number To Decimal String(number=w516) -> (decimal integer string=w517:string)  [unwired: 1 in]
            n367 = Number To Decimal String(number=w509) -> (decimal integer string=w514:string)  [unwired: 1 in]
            n368 = Get Date/Time String(date format (0)=enum16{"short", "long", "abbreviated"}."abbreviated", seconds (now)=w527, want seconds? (F)=TRUE) -> (time string=w518:string)  [unwired: 1 out]
            n369 = Bundle("PIEZO"=w522, "psd"=w515, "Z scanstart [nm]"=w521, "slope [nm/V]"=w520, "spring constant [N/m]"=w519, "pulling speed [nm/s]"=w516, "time string"=w518) -> (w508:T8)  [unwired: 1 in]
            n370 = Concatenate Strings(w524, w513, w517, "[nm_ s]", w513, w514) -> (w523:string)
            n371 = String To Path(string=w523) -> (path=w506:path)
            n372 = case shown="True" "to punias" {
              tunnel: w508 -> [_ w529]
              tunnel: w506 -> [_ w528]
              frame False {
              }
              frame True {
                n373 = call "punias_save.vi"("datalog path (use dialog)"=w528, "Cluster"=w529) -> ()  [unwired: 9 in, 1 out]
              }
            }
            n374 = case "datalog save" shown="True" "to datalog" {
              tunnel: "output folder" -> [_ w534]
              tunnel: w508 -> [_ w533]
              frame False {
              }
              frame True {
                n375 = call "XYsave.vi"("Cluster"=w533, "datalog path (use dialog)"=w534) -> ()  [unwired: 1 in, 2 out]
              }
            }
            n376 = case "txt save" shown="True" "to txt" {
              tunnel: w506 -> [_ w537]
              tunnel: w508 -> [_ w536]
              frame False {
              }
              frame True {
                n377 = call "XYsave_txt.vi"("Correct deflection"="deflection correction", "Cluster"=w536, "datalog path (use dialog)"=w537) -> ()  [unwired: 1 in, 1 out]
              }
            }
            "Boolean 2" <- TRUE ("Boolean 2")
          }
        }
      }
      frame "2" {
        n378 = flat-sequence {
          tunnel: w545 -> [w556]
          tunnel: w547 -> [w557]
          tunnel: w548 -> [w558]
          tunnel: w549 -> [w559]
          tunnel: w550 -> [w560]
          tunnel: w551 -> [w561]
          tunnel: w552 -> [w562]
          tunnel: [w562] -> w544
          tunnel: [w561] -> w543
          tunnel: [w560] -> w542
          tunnel: [w559] -> w541
          tunnel: [w558] -> w540
          tunnel: [w557] -> w539
          tunnel: [w556] -> w538
          tunnel: w544 -> [w597]
          tunnel: w543 -> [w596]
          tunnel: w542 -> [w592]
          tunnel: w541 -> [w591]
          tunnel: w540 -> [w589]
          tunnel: w539 -> [w585]
          tunnel: w538 -> [w572]
          frame #0 {
            n379 = local write "Boolean 2"(FALSE ("Boolean 2")) -> ()
            n380 = case shown="True" "autosave" {
              tunnel: [T7."IDLE" ("Enum 2") T7."SAVE" ("Enum 2")] -> w555
              frame False {
              }
              frame True {
              }
            }
            n381 = local write "state control"(w555) -> ()
          }
          frame #1 {
            n382 = local read "channels"() -> (w577:string[])
            n383 = call "disable-enable.vi"("Disabled"=T3."Disabled", "Array"=w592) -> ("error out"=w594:errorcluster)  [unwired: 1 in]
            n384 = Index Array(array=w577, index #1=1 ("index"), index #2=2 ("index"), index #3=3 ("index")) -> (element #1=w575:string, element #2=w574:string, element #3=w573:string)
            n385 = call "dynamika.vi"("error in"=w594, "dynamika [nm/s]"=w589, "scansize [nm]"=w597) -> ("error out"=w593:errorcluster, "czas trwania [s]"=w590:dbl)
            "pulling duration [s]" <- w590
            n386 = local read "output folder"() -> (w584:path)
            n387 = local read "accept calibration"() -> (w570:bool)
            n388 = Concatenate Strings(w575, ",", w574) -> (w576:string)
            n389 = call "trigen.vi"("piezo constant"=w572, "Invert?"=w596, "error in"=w593, "liczba probek"=w585, "scanstart [nm]"=w591, "scansize [nm]"=w597) -> ("error out"=w583:errorcluster, "Waveform Graph"=w582:dbl[])
            n390 = call "measure_cnt.vi"("error in (no error)"=w583, "datalog path (use dialog)"=w584) -> ("msr cnt"=→"curves count":dbl)  [unwired: 8 in, 1 out]
            n391 = call "VCmodule.vi"("input"=w576, "output"=w573, "signal"=w582, "piezo constant"=w572, "liczba probek"=w585, "czas trwania [s]"=w590) -> ("PIEZO"=w588:dbl[], "psd"=w587:dbl[])  [unwired: 1 out]
            n392 = case "correction" shown="True" w570 {
              tunnel: w588 -> [w599 w605]
              tunnel: [w599 w605] -> w586
              tunnel: [w600 w606] -> w569
              tunnel: w587 -> [w600 w607]
              tunnel: [0.0 ("spring constant [N/m]") "spring constant [N/m]"] -> w568
              frame False {
              }
              frame True {
                n393 = Multiply(x="spring constant [N/m]", y=1000.0) -> (x*y=w602:dbl)
                n394 = Multiply(x=w607, y="slope [nm/V]") -> (x*y=w608:dbl[])
                n395 = Multiply(x=w608, y=w602) -> (x*y=w606:dbl[])
              }
            }
            "psd" <- w569
            n396 = local read "RT DEFLECTION CORRECTION"() -> (w566:bool)
            n397 = call "poly_fit.vi"("liczba probek"=w585, "PIEZO"=w586) -> ("fitted piezo"=w565:dbl[])  [unwired: 9 in]
            "PIEZO" <- w565
            n398 = call "Deflection correction.vi"("fitted piezo"=w565, "psd"=w569, "spring constant [N/m]"=w568, "RT DEFLECTION CORRECTION"=w566) -> ("Array"=→"first":cluster{dbl[], dbl[]}[])  [unwired: 7 in]
          }
        }
        n399 = local read "state control"() -> (w546:T1)
      }
      frame "kalibracja" {
        n400 = flat-sequence {
          tunnel: [w622] -> w609
          tunnel: [w664] -> w610
          tunnel: w609 -> [w663]
          frame #0 {
            n401 = while {
              stop <- "stop 2" stop-if-true
              n402 = Wait (ms)(milliseconds to wait=u32 10) -> ()  [unwired: 1 out]
            }
            n403 = control-ref of="Boolean"() -> (w618:refnum<vi>)
            n404 = control-ref of="koniec"() -> (w615:refnum<vi>)
            n405 = control-ref of="ponów"() -> (w616:refnum<vi>)
            n406 = control-ref of="stop 2"() -> (w613:refnum<vi>)
            n407 = Build Array(w618, w615, w616) -> (w619:refnum<vi>[])
            n408 = call "disable-enable.vi"("Disabled"=T3."Disabled and Grayed Out", "Array"=w619) -> ("error out"=w614:errorcluster)  [unwired: 1 in]
            n409 = Build Array(w613) -> (w612:refnum<vi>[])
            n410 = call "disable-enable.vi"("error in (no error)"=w614, "Array"=w612) -> ()  [unwired: 1 in, 1 out]
            "Tab Control" <- enum32{"VELO", "KALIB", "channels"}."KALIB" ("Tab Control")
          }
          frame #1 {
            n411 = local read "channels"() -> (w626:string[])
            n412 = Index Array(array=w626, index=1) -> (element=w624:string)
            n413 = call "kalibracja_gensig.vi"("NI device/channel"=w624, "Averages"="Averages", "Sampling frequency [Hz]"="Sampling frequency [Hz]") -> ("error out"=w623:errorcluster, "mean"=w628:dbl, "Array"=w627:dbl[], "Spectrum Plot"=w629:cluster{dbl, "df":dbl, "Spectrum out":dbl[]})  [unwired: 1 in]
            n414 = case shown="No Error" w623 {
              tunnel: w629 -> [w652 _]
              tunnel: w623 -> [w649 _]
              tunnel: w628 -> [w646 _]
              tunnel: w627 -> [w645 _]
              tunnel: [FALSE ("true") w661] -> w622
              frame No Error {
                n415 = control-ref of="Boolean"() -> (w643:refnum<vi>)
                n416 = control-ref of="stop 2"() -> (w640:refnum<vi>)
                n417 = Build Array(w643) -> (w651:refnum<vi>[])
                n418 = call "disable-enable.vi"("error in (no error)"=w649, "Disabled"=T3."Enabled", "Array"=w651) -> ("error out"=w642:errorcluster)
                n419 = Build Array(w640) -> (w639:refnum<vi>[])
                n420 = call "disable-enable.vi"("error in (no error)"=w642, "Disabled"=T3."Disabled and Grayed Out", "Array"=w639) -> ("error out"=w641:errorcluster)
                n421 = while {
                  tunnel: [w658] -> w648
                  tunnel: [w657] -> w647
                  tunnel: w641 -> [w656]
                  tunnel: [w655] -> w644
                  stop <- "Boolean" stop-if-true
                  n422 = control-ref of="Spectrum Plot"() -> (w653:refnum<vi>)
                  n423 = property on="Property Node" class="WFGraph (strict)"(reference=w653, error in=w656, "Active Cursor"=1, "Active Cursor"=0) -> (error out=w655:errorcluster, "Cursor.Cursor Position:Cursor X"=w658:dbl, "Cursor.Cursor Position:Cursor X"=w657:dbl)  [unwired: 1 out]
                }
                n424 = control-ref of="koniec"() -> (w636:refnum<vi>)
                n425 = control-ref of="ponów"() -> (w635:refnum<vi>)
                n426 = Build Array(w636, w635) -> (w634:refnum<vi>[])
                n427 = call "kalibracja_powerpeak.vi"("mean"=w646, "error in"=w644, "Array"=w645, "Cursor.Cursor X"=w647, "Cursor.Cursor X 2"=w648) -> ("error out"=w637:errorcluster, "Est Power peak"=→"Est Power peak" →"power peak":dbl)  [unwired: 5 in]
                n428 = call "disable-enable.vi"("error in (no error)"=w637, "Array"=w634) -> ()  [unwired: 1 in, 1 out]
                "Spectrum Plot" <- w652
              }
              frame Error {
                n429 = One Button Dialog(message="Invalid device configuration!") -> (true=w661:bool)  [unwired: 1 in]
              }
            }
          }
          frame #2 {
            n430 = case shown="True" w663 {
              tunnel: [w665 T1."channels" ("state control")] -> w664
              frame False {
                n431 = while {
                  tunnel: ["ponów"] -> w666
                  stop <- w672 stop-if-true
                  n432 = Or(x="ponów", y="koniec") -> (x .or. y?=w672:bool)
                  n433 = Wait (ms)(milliseconds to wait=u32 10) -> ()  [unwired: 1 out]
                }
                n434 = case shown="False" w666 {
                  tunnel: [T7."IDLE" ("Enum 2") T7."kalibracja" ("Enum 2")] -> w665
                  frame False {
                    n435 = local write "Tab Control"(enum32{"VELO", "KALIB", "channels"}."VELO" ("Tab Control")) -> ()
                  }
                  frame True {
                  }
                }
              }
              frame True {
                n436 = local write "chnl_control"(enum16{"MAIN", "QUIT", "INIT", "SAVE"}."INIT" ("chnl_control")) -> ()
                n437 = local write "Tab Control"(enum32{"VELO", "KALIB", "channels"}."channels" ("Tab Control")) -> ()
              }
            }
          }
        }
      }
      frame "pad_cfg" {
        n438 = stacked-sequence "flatten sequence for better  readability" {
          seq-local: [w682 _ _ _] -> [_ w711 _ _]
          seq-local: [w681 _ _ _] -> [_ w715 _ _]
          seq-local: [_ w714 _ _] -> [_ _ w752 _]
          seq-local: [_ w713 _ _] -> [_ _ w751 _]
          seq-local: [_ w712 _ _] -> [_ _ w754 _]
          seq-local: [_ _ w752 _] -> [_ _ _ w778]
          seq-local: [_ _ w758 _] -> [_ _ _ w780]
          seq-local: [_ _ w757 _] -> [_ _ _ w781]
          seq-local: [_ _ w756 _] -> [_ _ _ w779]
          seq-local: [_ _ w755 _] -> [_ _ _ w777]
          seq-local: [_ _ w751 _] -> [_ _ _ w776]
          frame #0 {
            n439 = call "current_folder.vi"("filename"="\\config") -> ("Path"=w678:path)  [unwired: 10 in]
            n440 = call <vilib>:"Check if File or Folder Exists.vi"("path"=w678) -> ("error out"=w683:errorcluster, "file or folder exists?"=w684:bool, "dup path"=w679:path)  [unwired: 8 in]
            n441 = case shown="True" w684 {
              tunnel: [TRUE w696] -> w685
              tunnel: [w690 w693] -> w686
              tunnel: w683 -> [w688 w694]
              tunnel: w679 -> [w687 w692]
              frame False {
                n442 = Open/Create/Replace File(file path (use dialog)=w687, error in=w688, operation (0:open)=T2."create") -> (error out=w690:errorcluster)  [unwired: 3 in, 2 out]
              }
              frame True {
                n443 = Get File Size(file=w692, error in=w694) -> (size (in bytes)=w695:i64, 0:w693:errorcluster)  [unwired: 1 out]
                n444 = Less?(x=w695, y=i64 10) -> (x < y?=w696:bool)
              }
            }
            n445 = case shown="True" w685 {
              tunnel: w678 -> [w698 w700]
              tunnel: w686 -> [w699 w702]
              tunnel: [w699 w701] -> w681
              tunnel: [w698 w700] -> w682
              frame False {
              }
              frame True {
                n446 = for {
                  N: 14 -> [_]
                  tunnel: [w708] -> w703 mode=indexing
                  i -> [w706]
                  n447 = Increment(x=w706) -> (x+1=w705:i32)
                  n448 = Number To Hexadecimal String(2:w705) -> (0:w709:string)  [unwired: 1 in]
                  n449 = Concatenate Strings("0" ("string"), w709) -> (w708:string)
                }
                n450 = Write to Text File(file (use dialog)=w700, text=w703, error in=w702) -> (error out=w701:errorcluster)  [unwired: 1 in, 2 out]
              }
            }
          }
          frame #1 {
            w718 = FALSE ("Boolean")
            n451 = Read from Text File(file (use dialog)=w711, error in=w715) -> (refnum out=w736:refnum<file>, text=w743:string, error out=w737:errorcluster)  [unwired: 2 in, 1 out]
            n452 = call-poly <vilib>:"Read From Spreadsheet File.vi"("format (%d)"="%x", "file path (dialog if empty)"=w711) -> ("all rows"=w720:i64[][])  [unwired: 5 in, 4 out]
            n453 = Build Array(w718, w718, w718, w718, w718, w718, w718, w718, w718, w718, w718, w718) -> (→"appended array":bool[])
            n454 = Close File(refnum=w736, error in=w737) -> (path=w714:path, error out=w735:errorcluster)
            n455 = Reshape Array(w720, 14 ("dimension size")) -> (→"read":i64[])
            n456 = control-ref of="Ring"() -> (w734:refnum<vi>)
            n457 = control-ref of="Ring 2"() -> (w733:refnum<vi>)
            n458 = control-ref of="Ring 3"() -> (w732:refnum<vi>)
            n459 = control-ref of="Ring 4"() -> (w731:refnum<vi>)
            n460 = control-ref of="Ring 5"() -> (w730:refnum<vi>)
            n461 = control-ref of="Ring 6"() -> (w729:refnum<vi>)
            n462 = control-ref of="Ring 7"() -> (w728:refnum<vi>)
            n463 = control-ref of="Ring 8"() -> (w727:refnum<vi>)
            n464 = control-ref of="Ring 9"() -> (w726:refnum<vi>)
            n465 = control-ref of="Ring 10"() -> (w725:refnum<vi>)
            n466 = control-ref of="Ring 11"() -> (w724:refnum<vi>)
            n467 = control-ref of="Ring 12"() -> (w723:refnum<vi>)
            n468 = control-ref of="Ring 13"() -> (w722:refnum<vi>)
            n469 = control-ref of="Ring 14"() -> (w721:refnum<vi>)
            n470 = Spreadsheet String To Array(delimiter (Tab)="\\n", format string="%x", spreadsheet string=w743, array type (2D Dbl)=0) -> (array=w741:i32[][])
            n471 = Build Array(w734, w733, w732, w731, w730, w729, w728, w727, w726, w725, w724, w723, w722, w721) -> (w713:refnum<vi>[])
            n472 = Reshape Array(w741, 14 ("dimension size")) -> (w738:i32[])
            n473 = for {
              tunnel: w713 -> [w745] mode=indexing
              tunnel: w738 -> [w750] mode=indexing
              tunnel: w735 -> [w747]
              tunnel: [w746] -> w712
              n474 = property class="Ring (strict)"(reference=w745, error in=w747, "Value"=w750) -> (reference out=w749:refnum<vi>, error out=w748:errorcluster)
              n475 = Close Reference(reference=w749, error in (no error)=w748) -> (error out=w746:errorcluster)
            }
          }
          frame #2 {
            n476 = control-ref of="gpd_confirm"() -> (w765:refnum<vi>)
            n477 = property class="Bool"(reference=w765, error in=w754, "DisabledEnum"=T3."Disabled and Grayed Out" ("Disabled")) -> (reference out=w766:refnum<vi>, error out=w767:errorcluster)
            n478 = call <vilib>:"Query Input Devices.vi"("error in (no error)"=w767) -> ("error out"=w762:errorcluster, "joystick info"=w763:T9)  [unwired: 7 in, 2 out]
            n479 = while {
              tunnel: [w774] -> w756
              tunnel: ["index"] -> w757
              tunnel: [w769] -> w753
              tunnel: [w771] -> w758
              tunnel: w763 -> [w770]
              tunnel: w762 -> [w769]
              stop <- "device_ok" stop-if-true
              n480 = Index Array(array=w770, index="index") -> (element=w775:T10)
              n481 = Unbundle(w775) -> ("axes total"=w774:u32, "buttons total"=w771:u32, "device name"=→"device name":string)  [unwired: 1 out]
            }
            n482 = property class="Bool"(reference=w766, error in=w753, "DisabledEnum"=T3."Enabled" ("Disabled")) -> (reference out=w761:refnum<vi>, error out=w760:errorcluster)
            n483 = Close Reference(reference=w761, error in (no error)=w760) -> (error out=w755:errorcluster)
          }
          frame #3 {
            n484 = Greater Or Equal?(x=w780, y=u32 10) -> (x >= y?=w785:bool)
            n485 = call <vilib>:"Initialize Joystick.vi"("error in (no error)"=w777, "device index"=w781) -> ("error out"=w783:errorcluster, "device ID"=w782:refnum<k1>)  [unwired: 8 in]
            n486 = case shown="True" w785 {
              tunnel: w779 -> [_ w793]
              tunnel: w782 -> [_ w792]
              tunnel: w783 -> [_ w791]
              tunnel: w778 -> [_ w790]
              tunnel: w776 -> [_ w789]
              frame False {
                n487 = One Button Dialog(message="002\nYou need at least 10 buttons") -> ()  [unwired: 1 in, 1 out]
                n488 = local write "state control"(T1."INIT" ("state control")) -> ()
                n489 = local write "Tab Control"(enum32{"VELO", "KALIB", "channels", "gamepad"}."VELO" ("Tab Control")) -> ()
              }
              frame True {
                n490 = while {
                  tunnel: w793 -> [w803]
                  tunnel: w792 -> [w801]
                  tunnel: w791 -> [w800]
                  tunnel: w790 -> [w796]
                  tunnel: w789 -> [w794]
                  stop <- w795 stop-if-true
                  n491 = call-poly <vilib>:"Acquire Input Data.vi"("device ID"=w801, "error in (no error)"=w800) -> ("button info"=w802:T11, "direction info"=w799:T12, "error out"=w798:errorcluster)  [unwired: 13 in, 2 out]
                  n492 = Wait Until Next ms Multiple(millisecond multiple=u32 25) -> ()  [unwired: 1 out]
                  n493 = case shown="No Error" w798 {
                    tunnel: w803 -> [_ _]
                    tunnel: w802 -> [w858 _]
                    tunnel: w799 -> [w857 _]
                    tunnel: w796 -> [w806 _]
                    tunnel: [w805 TRUE] -> w795
                    tunnel: w794 -> [w804 _]
                    frame No Error {
                      n494 = Unbundle By Name(w857) -> ("pov 1"=w852:i32)
                      n495 = case shown="True" "gpd_confirm" {
                        tunnel: w806 -> [_ w864]
                        tunnel: [FALSE TRUE] -> w805
                        tunnel: w804 -> [_ w860]
                        frame False {
                        }
                        frame True {
                          n496 = for {
                            N: 14 -> [_]
                            tunnel: [w876] -> w867 mode=indexing
                            tunnel: [w871] -> w865
                            tunnel: w860 -> [w870] mode=indexing
                            n497 = property class="Ring (strict)"(reference=w870) -> (reference out=w873:refnum<vi>, error out=w872:errorcluster, "Value"=w874:u16)  [unwired: 1 in]
                            n498 = Close Reference(reference=w873, error in (no error)=w872) -> (error out=w871:errorcluster)
                            n499 = Number To Hexadecimal String(2:w874) -> (0:w877:string)  [unwired: 1 in]
                            n500 = Concatenate Strings("0" ("string"), w877) -> (w876:string)
                          }
                          n501 = local write "state control"(T1."INIT" ("state control")) -> ()
                          n502 = local write "Tab Control"(enum32{"VELO", "KALIB", "channels", "gamepad"}."VELO" ("Tab Control")) -> ()
                          n503 = Write to Text File(file (use dialog)=w864, text=w867, error in=w865) -> (refnum out=w869:refnum<file>, error out=w868:errorcluster)  [unwired: 1 in, 1 out]
                          n504 = Close File(refnum=w869, error in=w868) -> ()  [unwired: 2 out]
                        }
                      }
                      n505 = Equal?(x=w852, y=0) -> (x = y?=w824:bool)
                      "pov 1" <- w824
                      n506 = Equal?(x=w852, y=90) -> (x = y?=w827:bool)
                      "pov 4" <- w827
                      n507 = Equal?(x=w852, y=270) -> (x = y?=w825:bool)
                      "pov 2" <- w825
                      n508 = Equal?(x=w852, y=180) -> (x = y?=w826:bool)
                      "pov 3" <- w826
                      n509 = Unbundle By Name(w858) -> ("button 1"=w850:bool, "button 2"=w849:bool, "button 3"=w846:bool, "button 4"=w844:bool, "button 5"=w842:bool, "button 6"=w841:bool, "button 7"=w839:bool, "button 8"=w837:bool, "button 9"=w835:bool, "button 10"=w833:bool)
                      "button 1" <- w850
                      "button 2" <- w849
                      "button 3" <- w846
                      "button 4" <- w844
                      "button 5" <- w842
                      "button 6" <- w841
                      "button 7" <- w839
                      "button 8" <- w837
                      "button 9" <- w835
                      "button 10" <- w833
                      n510 = feedback-in #1(w850) -> ()
                      n511 = feedback #1() -> (w851:bool)  [unwired: 1 in]
                      n512 = feedback #2() -> (w848:bool)  [unwired: 1 in]
                      n513 = feedback-in #2(w849) -> ()
                      n514 = feedback #3() -> (w847:bool)  [unwired: 1 in]
                      n515 = feedback-in #3(w846) -> ()
                      n516 = feedback #4() -> (w845:bool)  [unwired: 1 in]
                      n517 = feedback-in #4(w844) -> ()
                      n518 = feedback #5() -> (w843:bool)  [unwired: 1 in]
                      n519 = feedback-in #5(w842) -> ()
                      n520 = feedback #6() -> (w840:bool)  [unwired: 1 in]
                      n521 = feedback-in #6(w841) -> ()
                      n522 = feedback #7() -> (w838:bool)  [unwired: 1 in]
                      n523 = feedback-in #7(w839) -> ()
                      n524 = feedback #8() -> (w836:bool)  [unwired: 1 in]
                      n525 = feedback-in #8(w837) -> ()
                      n526 = feedback #9() -> (w834:bool)  [unwired: 1 in]
                      n527 = feedback-in #9(w835) -> ()
                      n528 = feedback #10() -> (w832:bool)  [unwired: 1 in]
                      n529 = feedback-in #10(w833) -> ()
                      n530 = feedback #11() -> (w831:bool)  [unwired: 1 in]
                      n531 = feedback-in #11(w824) -> ()
                      n532 = feedback #12() -> (w830:bool)  [unwired: 1 in]
                      n533 = feedback-in #12(w825) -> ()
                      n534 = feedback #13() -> (w829:bool)  [unwired: 1 in]
                      n535 = feedback-in #13(w826) -> ()
                      n536 = feedback #14() -> (w828:bool)  [unwired: 1 in]
                      n537 = feedback-in #14(w827) -> ()
                      n538 = Exclusive Or(1:w851, 2:w850) -> (0:w823:bool)
                      n539 = Exclusive Or(1:w848, 2:w849) -> (0:w822:bool)
                      n540 = Exclusive Or(1:w847, 2:w846) -> (0:w821:bool)
                      n541 = Exclusive Or(1:w844, 2:w845) -> (0:w820:bool)
                      n542 = Exclusive Or(1:w842, 2:w843) -> (0:w819:bool)
                      n543 = Exclusive Or(1:w840, 2:w841) -> (0:w818:bool)
                      n544 = Exclusive Or(1:w839, 2:w838) -> (0:w817:bool)
                      n545 = Exclusive Or(1:w836, 2:w837) -> (0:w816:bool)
                      n546 = Exclusive Or(1:w834, 2:w835) -> (0:w815:bool)
                      n547 = Exclusive Or(1:w832, 2:w833) -> (0:w814:bool)
                      n548 = Exclusive Or(1:w824, 2:w831) -> (0:w813:bool)
                      n549 = Exclusive Or(1:w825, 2:w830) -> (0:w812:bool)
                      n550 = Exclusive Or(1:w826, 2:w829) -> (0:w811:bool)
                      n551 = Exclusive Or(1:w827, 2:w828) -> (0:w810:bool)
                      n552 = Build Array(w823, w822, w821, w820, w819, w818, w817, w816, w815, w814, w813, w812, w811, w810) -> (w809:bool[])
                      n553 = for {
                        N: 14 -> [_]
                        tunnel: w809 -> [w879] mode=indexing
                        i -> [w878]
                        n554 = case shown="True" w879 {
                          tunnel: w878 -> [_ w885]
                          frame False {
                          }
                          frame True {
                            n555 = local read "appended array"() -> (w883:bool[])
                            n556 = local read "read"() -> (w884:i64[])
                            n557 = Index Array(array=w884, index=w885) -> (element=w882:i64)
                            n558 = Index Array(array=w883, index=w882) -> (element=w881:bool)
                            n559 = Not(x=w881) -> (.not. x?=w880:bool)
                            n560 = Delete From Array(array=w883, length=1, index=w882) -> (array with subset deleted=w887:bool[])  [unwired: 1 out]
                            n561 = Insert Into Array(array=w887, index=w882, new element=w880) -> (w886:bool[])
                            n562 = local write "appended array"(w886) -> ()
                          }
                        }
                      }
                    }
                    frame Error {
                      n563 = One Button Dialog(message="001\nDevice not plugged or not selected.\nIf device is freshly detected, restart is required.") -> ()  [unwired: 1 in, 1 out]
                    }
                  }
                }
              }
            }
            "device index" <- w781
          }
        }
      }
      frame "channels" {
        n564 = while {
          stop <- w895 stop-if-true
          n565 = local read "chnl_control"() -> (w892:enum16{"MAIN", "QUIT", "INIT", "SAVE"})
          n566 = case shown="\"SAVE\"" w892 {
            tunnel: [enum16{"MAIN", "QUIT", "INIT", "SAVE"}."MAIN" ("Enum") w919 enum16{"MAIN", "QUIT", "INIT", "SAVE"}."INIT" ("Enum") enum16{"MAIN", "QUIT", "INIT", "SAVE"}."QUIT" ("Enum")] -> w893
            frame "INIT" {
              n567 = call "current_folder.vi"("extension"=".txt" ("string"), "filename"="\\channel_ini" ("string")) -> ("Path"=w901:path)  [unwired: 9 in]
              "path" <- w901
              n568 = call <vilib>:"Check if File or Folder Exists.vi"("path"=w901) -> ("error out"=w898:errorcluster, "file or folder exists?"=w900:bool, "dup path"=w899:path)  [unwired: 8 in]
              n569 = case shown="True" w900 {
                tunnel: w899 -> [_ w915]
                tunnel: w898 -> [w907 w914]
                tunnel: [w907 w914] -> w897
                frame False {
                }
                frame True {
                  n570 = control-ref of="[(A+B)-(C+D)]/(A+B+C+D)"() -> (w912:refnum<vi>)
                  n571 = control-ref of="A+B+C+D"() -> (w911:refnum<vi>)
                  n572 = control-ref of="PIEZO INPUT"() -> (w913:refnum<vi>)
                  n573 = control-ref of="PIEZO OUTPUT"() -> (w908:refnum<vi>)
                  n574 = Build Array(w911, w912, w913, w908) -> (w910:refnum<vi>[])
                  n575 = call-poly <vilib>:"Read From Spreadsheet File.vi"("file path (dialog if empty)"=w915) -> ("all rows"=w909:string[][])  [unwired: 6 in, 4 out]
                  n576 = for {
                    tunnel: w910 -> [w918] mode=indexing
                    tunnel: w909 -> [w917] mode=indexing
                    n577 = Index Array(array=w917) -> (element=w916:string)  [unwired: 1 in]
                    n578 = property class="DAQmxName"(reference=w918, "Value"=w916) -> ()  [unwired: 1 in, 2 out]
                  }
                }
              }
              n579 = case shown="Error" w897 {
                selector: w897 -> [_ w906]
                frame No Error {
                }
                frame Error {
                  n580 = call <vilib>:"Clear Errors.vi"("error in (no error)"=w906) -> ()  [unwired: 6 in, 1 out]
                  n581 = One Button Dialog(message="Error occured during creating a new file.") -> (true=w904:bool)  [unwired: 1 in]
                  n582 = Stop(stop? (T)=w904) -> ()
                }
              }
            }
            frame "MAIN" {
              n583 = while {
                tunnel: [w921] -> w919
                stop <- w920 stop-if-true
                n584 = event shown="[0] \"SAVE 2\": Value Change" {
                  selector: _ -> [_ _ _]
                  dyn-events: _ -> [_ _ _]
                  timeout: _ -> [_ _ _]
                  tunnel: [enum16{"MAIN", "QUIT", "INIT", "SAVE"}."SAVE" ("Enum") enum16{"MAIN", "QUIT", "INIT", "SAVE"}."INIT" ("Enum") enum16{"MAIN", "QUIT", "INIT", "SAVE"}."QUIT" ("Enum")] -> w921
                  tunnel: [TRUE TRUE TRUE] -> w920
                  event "SAVE 2": Value Change {
                    n585 = event-data() -> ()  [unwired: 1 in, 6 out]
                  }
                  event "RELOAD CONFIG": Value Change {
                    n586 = event-data() -> ()  [unwired: 1 in, 6 out]
                  }
                  event "QUIT": Value Change {
                    n587 = event-data() -> ()  [unwired: 1 in, 6 out]
                    n588 = case shown="True" "QUIT" {
                      frame False {
                      }
                      frame True {
                        n589 = local write "state control"(T6."INIT" ("state control")) -> ()
                        n590 = local write "Tab Control"(enum32{"VELO", "KALIB", "channels"}."VELO" ("Tab Control")) -> ()
                      }
                    }
                  }
                }
              }
            }
            frame "SAVE" {
              n591 = flat-sequence {
                tunnel: [w935] -> w932
                tunnel: [w937] -> w934
                tunnel: [w938] -> w933
                tunnel: w932 -> [w937]
                tunnel: w934 -> [w948]
                tunnel: w933 -> [w947]
                frame #0 {
                  n592 = local read "path"() -> (w935:path)
                  n593 = Open/Create/Replace File(file path (use dialog)=w935, operation (0:open)=T2."replace or create") -> ()  [unwired: 4 in, 3 out]
                }
                frame #1 {
                  w939 = "\r\n"
                  n594 = Concatenate Strings("A+B+C+D", w939, "[(A+B)-(C+D)]/(A+B+C+D)", w939, "PIEZO INPUT", w939, "PIEZO OUTPUT") -> (w940:string)
                  n595 = Write to Text File(file (use dialog)=w937, text=w940) -> (refnum out=w941:refnum<file>, error out=w942:errorcluster)  [unwired: 2 in, 1 out]
                  n596 = Close File(refnum=w941, error in=w942) -> (error out=w938:errorcluster)  [unwired: 1 out]
                }
                frame #2 {
                  n597 = while {
                    tunnel: w948 -> [w951]
                    tunnel: w947 -> [w950]
                    stop <- w949 stop-if-true
                    n598 = call <vilib>:"Check if File or Folder Exists.vi"("error in (no error)"=w950, "path"=w951) -> ("file or folder exists?"=w949:bool)  [unwired: 7 in, 2 out]
                  }
                }
              }
            }
            frame "QUIT" {
            }
          }
          n599 = Equal?(x=enum16{"MAIN", "QUIT", "INIT", "SAVE"}."QUIT" ("Enum"), y=w892) -> (x = y?=w895:bool)
          n600 = local write "chnl_control"(w893) -> ()
        }
        n601 = local read "state control"() -> (w891:T1)
      }
    }
  }
